vi "Base GEA3 Tool.vi"() -> ()   [LabVIEW 2021]
uses:
  Common/LabVIEW GEA2 Toolkit/GEA3/type defs/Data In.ctl
  Common/LabVIEW GEA2 Toolkit/GEA3/type defs/Source_Destination.ctl
  Common/LabVIEW GEA2 Toolkit/GEA3/type defs/ERD Write Data In.ctl
  Common/LabVIEW GEA2 Toolkit/GEA3/type defs/Data Type.ctl
  Common/LabVIEW GEA2 Toolkit/GEA3/type defs/ERD Read Data Out.ctl
  Common/LabVIEW GEA2 Toolkit/GEA3/type defs/ERD Read Data In.ctl
  Dryer Tool (Commercial 2)/JL Dryer Tool Support/type defs/Programming.ctl
  Dryer Tool (Commercial 2)/JL Dryer Tool Support/type defs/Flash_Results.ctl
  Dryer Tool (Commercial 2)/JL Dryer Tool Support/type defs/ERD_Always_Show_JL.ctl
  Common/GEA2 Script/typedefs/Script Info.ctl
  <vilib>/Platform/fileVersionInfo.llb/FileVersionInformation.ctl
  Dryer Tool (Commercial 2)/JL Dryer Tool Support/type defs/Choose_ERD_List.ctl
  Common/Diagnostics Decode/Type Defs/Diag_FaultTableStatus.ctl
  Common/Diagnostics Decode/Type Defs/Diag_FaultTableEntry.ctl
  Common/Diagnostics Decode/Type Defs/Diag_EntityManifestType.ctl
  Common/Diagnostics Decode/Type Defs/Diag_FaultSeqEntry.ctl
  Automation2/Product Specific/Clothes Care/Justice League/Product Testcode/Diagnostics/TypeDefs/Centauro Diagnostic V3 SnapShot.ctl
  Dryer Tool (Commercial 2)/JL Dryer Tool Support/type defs/JL_Diagnost V3 Cycle History.ctl
  Dryer Tool (Commercial 2)/JL Dryer Tool Support/type defs/ERDList.ctl
  Dryer Tool (Commercial 2)/JL Dryer Tool Support/type defs/ERD_Loop_States_JL.ctl
  Dryer Tool (Commercial 2)/JL Dryer Tool Support/type defs/Version.ctl
  Dryer Tool (Commercial 2)/JL Dryer Tool Support/type defs/BootloaderVersion.ctl
  Common/LabVIEW GEA2 Toolkit/GEA3/type defs/Data Out.ctl
  D:/Common/LabVIEW GEA2 Toolkit/source/GEA3 DLL Source/GeaCommunication.dll
  Common/LabVIEW GEA2 Toolkit/source/GEA3 DLL Source/GeaCommunication.dll
  Common/GExplorer Support/typedefs/GExplorer_Data_Cluster.ctl
  Dryer Tool (Commercial 2)/JL Dryer Tool Support/type defs/ERD_Data_Loop_Control.ctl
  Dryer Tool (Commercial 2)/JL Dryer Tool Support/type defs/Error_Command.ctl
  Dryer Tool (Commercial 2)/JL Dryer Tool Support/type defs/Cont_Send_States.ctl
  Dryer Tool (Commercial 2)/JL Dryer Tool Support/type defs/All_Bundled_Data_JL.ctl
  Dryer Tool (Commercial 2)/JL Dryer Tool Support/type defs/CSV_File_String_Arrays.ctl
  Dryer Tool (Commercial 2)/JL Dryer Tool Support/type defs/Fault Table Array.ctl
  Dryer Tool (Commercial 2)/JL Dryer Tool Support/type defs/Fault_Table_Info.ctl
  Dryer Tool (Commercial 2)/JL Dryer Tool Support/type defs/Heat Control.ctl
  Dryer Tool (Commercial 2)/JL Dryer Tool Support/type defs/ERD_Commercial_Laundry.ctl
  Dryer Tool (Commercial 2)/JL Dryer Tool Support/type defs/ERD_RJ45.ctl
  Dryer Tool (Commercial 2)/JL Dryer Tool Support/type defs/DAQ_Control_Command.ctl
  Dryer Tool (Commercial 2)/JL Dryer Tool Support/type defs/ERD_Loop_Control_Command.ctl
  Dryer Tool (Commercial 2)/JL Dryer Tool Support/type defs/GEA2_Control_Command.ctl
  Common/LabVIEW GEA2 Toolkit/GEA3/advanced/GEA2 Message Received Event Handler.vi
  Common/LabVIEW GEA2 Toolkit/GEA3/library/GEA2_Toolkit.lvlib
panel:
  out "Message":string
  in  "EndOfCycle":bool
  in  "Board Index":u8=1 min=3 max=10 step=1
  in  "Pause(mls)":u32=100
  out "Rate":u32=100
  out "State":T1=enum."Read ERDs"
  out "ERD_Always Show":T2={"Inlet Thermistor"=0, "Machine State"="IDLE", "Filtered Moisture"=0, "Cycle Selected"="", "HTR 1 / Inner / Top"=FALSE, "HTR 2 / Outer / Bot"=FALSE, "Door Switch"=FALSE, "Drum Light"=FALSE, "Cycle Engine State"="", "Centrifugal Switch"=FALSE, "Drum Motor"=FALSE, "Cycle Count"=0, "Ext. Tumble"=FALSE, "eDry"=FALSE, "Temp Level"="", "Dryness Level"="", "Time Level"="", "Delay Time (min)"=0, "Steam Refresh"=FALSE, "Damp Alert"=FALSE, "Sub-Cycle"="", "Outlet Thermistor"=0, "Target Moisture"=0, "Remaining Cycle Time"=0, "Raw Moisture"=0, "Cycle Name"="", "My Cycle"=FALSE, "Delay Dry"=FALSE, "Detangle"=FALSE, "Control Lock"=FALSE, "Steam Valve"=FALSE, "Door Latch"=FALSE, "Signal Volume"="", "Tune ID"="", "Restr Detect Status"="", "Vent Restriction"="", "Load Size by Contact"="", "Load Size by Temp"="", "EOC Reason"="", "Sensor Dry Status"="", "Dampness State"="", "Target Voltage Reached"=FALSE, "TrimInhibitR1"=FALSE, "TrimInhibitR2"=FALSE, "TrimBothCoilInhibit"=FALSE, "NormalHeatControl"=FALSE, "HeatControl Request"=FALSE, "Cool Down Status"="", "EcoDryInhibitRelay1"=FALSE, "EcoDryInhibitRelay2"=FALSE, "ReverseDrumInhibitRelay1"=FALSE, "ReverseDrumInhibitRelay2"=FALSE, "OverTempHeaterInhibitRequest"=FALSE, "FallbackHeatControlMethodStatus"=FALSE, "IHC TimeSeconds"=0, "ECT TimeSeconds "=0, "SC Total Drying Time(S')"=0, "TTR Target Voltage (S')"=0, "TCT Drying Time (S's)"=0, "Drum Motor State"=enum."Off", "Load Size by Ag"="", "MaxFIletered Voltage"=0, "Dry Load Detection"="", "Min Sensing Elapse Sec"=0, "Time Multi Sec X100"=0, "Time Adder  Sec"=0, "Temp Multi EcoDry"="", "Temp Multi ExtraLow"="", "Temp Multi Low "="", "Temp Multi Medium"="", "Temp Multi High"="", "SmoothMoisture"=0, "Eco Dry SEL Status"="", "Eco Dry SEL Result"="", "Eco Dry Cont Status"="", "Eco Dry Relay1 Timer"="", "Eco Dry Relay2 Timer "="", "Eco Dry Stage 2 Tans "=0, "WiFiCommissioningPSt"="IDLE", "Payment Method"=""}
  out "Temp ADC":T3
  in  "Read Parametric":bool=TRUE
  in  "Data ON":bool=TRUE
  in  "Stop":bool
  in  "Reset":bool
  in  "UI Launch":bool
  in  "Tab Control":T4(tab)=enum."ERD List"
  out "Personality Set":u8=1
  in  "?":u8=1
  in  "Set Personality":bool
  out "CSV File Log Path":path=path "D:/QA/Commercial 2/Dryer_Xolo/ProbandoC2_24-11-21_15-05-37.csv"
  out "Version":T5
  in  "Read ERD List":T6[](array[typedef])=[{"ERD Number"=49, "Data Type"=enum."string"}] {"ERD Number" format="%.0x"}
  in  "Read ERD":bool
  in  "Write ERD List":T7[](array[typedef])=[{"ERD Number"=49, "Data Type"=enum."string", "Data"="01"}] {"ERD Number" format="%.0x"}
  in  "Write ERD":bool
  out "Read ERD Data Out":T9[](array[typedef])=[{"ERD Number"=49, "Data"="00 00 00 16"}] {"ERD Number" format="%.0x"}
  out "Boot Loader Version":T10
  in  "GEA Inputs":T11={"Source"=229, "Destination"=192} {"Destination" format="%.0x"; "Source" format="%.0x"}
  out "OK?":bool
  in  "Parametric":T12(ring)
  in  "Exit Botloader":bool
  in  "Enum":enum16{"All", "MC", "UI"}(ring)
  in  "Entry Botloader":bool
  out "FileVersionInfo":T13
  out "LabView/Version Number":string
  in  "Tool Version":bool=TRUE
  out "GEA2 Log":string
  in  "Save Log":bool
  in  "GEA2 Log Length":i32=100000
  in  "Clear":bool
  in  "Ignore this CMD":string
  in  "Filter Data":bool=TRUE
  in  "Programming":T14={"Program"=FALSE, "File Path"=path "", "Program Ind"=FALSE, "Reset Board"=FALSE, "Enter Bootloader"=FALSE, "Result"=9} {"Result" items=["ImageRejected", "BoardNotFound", "UnableToGetGeaConfiguration", "WriteToFlashNotAllowed", "ImageDownloadedSuccessfully", "ImagePresent", "WriteToFlashFailed", "EraseFailed", "CrcFailed", ""]}
  in  "Flash Latest":bool
  in  "Send Button":bool
  in  "GEA2 Send":T16={"Source"=228, "Destination"=192, "Command"=0, "Message"=""} {"Command" format="%02x"; "Destination" format="%02x"; "Source" format="%02x"}
  in  "Msg Rate (ms)":u32=1000 min=50 step=50
  in  "Start Send":bool
  out "Converted Data Out":T17 {"CRC" format="%04x"; "Length" format="%02x"; "Command" format="%02x"; "Destination" format="%02x"; "Source" format="%02x"}
  in  "Write parametric":bool
  in  "Message to send":string="04 03"
  in  "Get Faults":bool
  in  "Clear Fault Table Buffer":bool
  in  "Clear Fault Seq Buffer":bool
  out "Fault Sequence Entries":T18[](array[typedef])
  out "Fault Seq Status":T19
  out "Fault Table Entries":T20[](array[typedef])
  out "Fault Table Status":T19
  out "Diagnostic Entity Manifest":T21
  out "Major Version":u8
  out "Minor Version":u8
  out "Fault Set?":bool
  in  "Filter by Count":bool=TRUE
  out "Centauro Fault Snapshot":T22
  in  "ERD Spam GEA Inputs":T11={"Source"=229, "Destination"=192} {"Destination" format="%.0x"; "Source" format="%.0x"}
  in  "Get Cycle Data":bool
  in  "Filter by Status Count":bool=TRUE
  out "JL Cycle History":T23
  out "output cluster":T19
  in  "Script Log Path":path
  in  "Run Script":bool
  out "Script Pass/Fail?":bool
  out "Script Report Text":string
  in  "stop script":bool
  in  "Script Path":path
  out "Script Info":T24 {"Overall Script File Progress" scale=0.0..1.0; "Elapsed time (s)" format="%#.1f"; "Current Script Progress" scale=0.0..1.0}
  out "Script Error Out":errorcluster
  in  "Load ERD List":T25
  in  "ERD Default List":T26 {"ERD Number" format="%x"}
  in  "ERD's List Ticket Testing":T26 {"ERD Number" format="%x"}
  in  "Wifi State":T27(ring)
  in  "Set Wifi State(ERD 6003)":bool
  in  "Turn on Wifi":bool
  in  "Turn off Wifi":bool
  out "Wifi Network State":string
  out "Wifi Password":string
  out "Wifi Network Name":string
  out "Mac Address":string
  in  "Get Wifi Data":bool
  out "Error Out":errorcluster
  # "Personality"
  # "Ver. 1.3"
  # "This controls destination of ERD Spam.\nYou should never change source unless\nyou want to see the spam in the GEA log."
  # "Wifi State is Writing to ERD 6003 and communicating with the wifi board directly.  It will remain in the state you wrote it to until another command is recieved. \n\nOnly Write to invalid if you are testing the board in Invalid state."
  # "After turning on Wifi , wait about 30 seconds and press the Get Wifi Data button.  Network state should be 1, apmode.\n\nAll this is doing is Writing the ERD 0xF115 Service Request to request connect, or disconnect."
  # "Contact:\n\nTerrance Bradford\nTerrance.Bradford@geappliances.com"
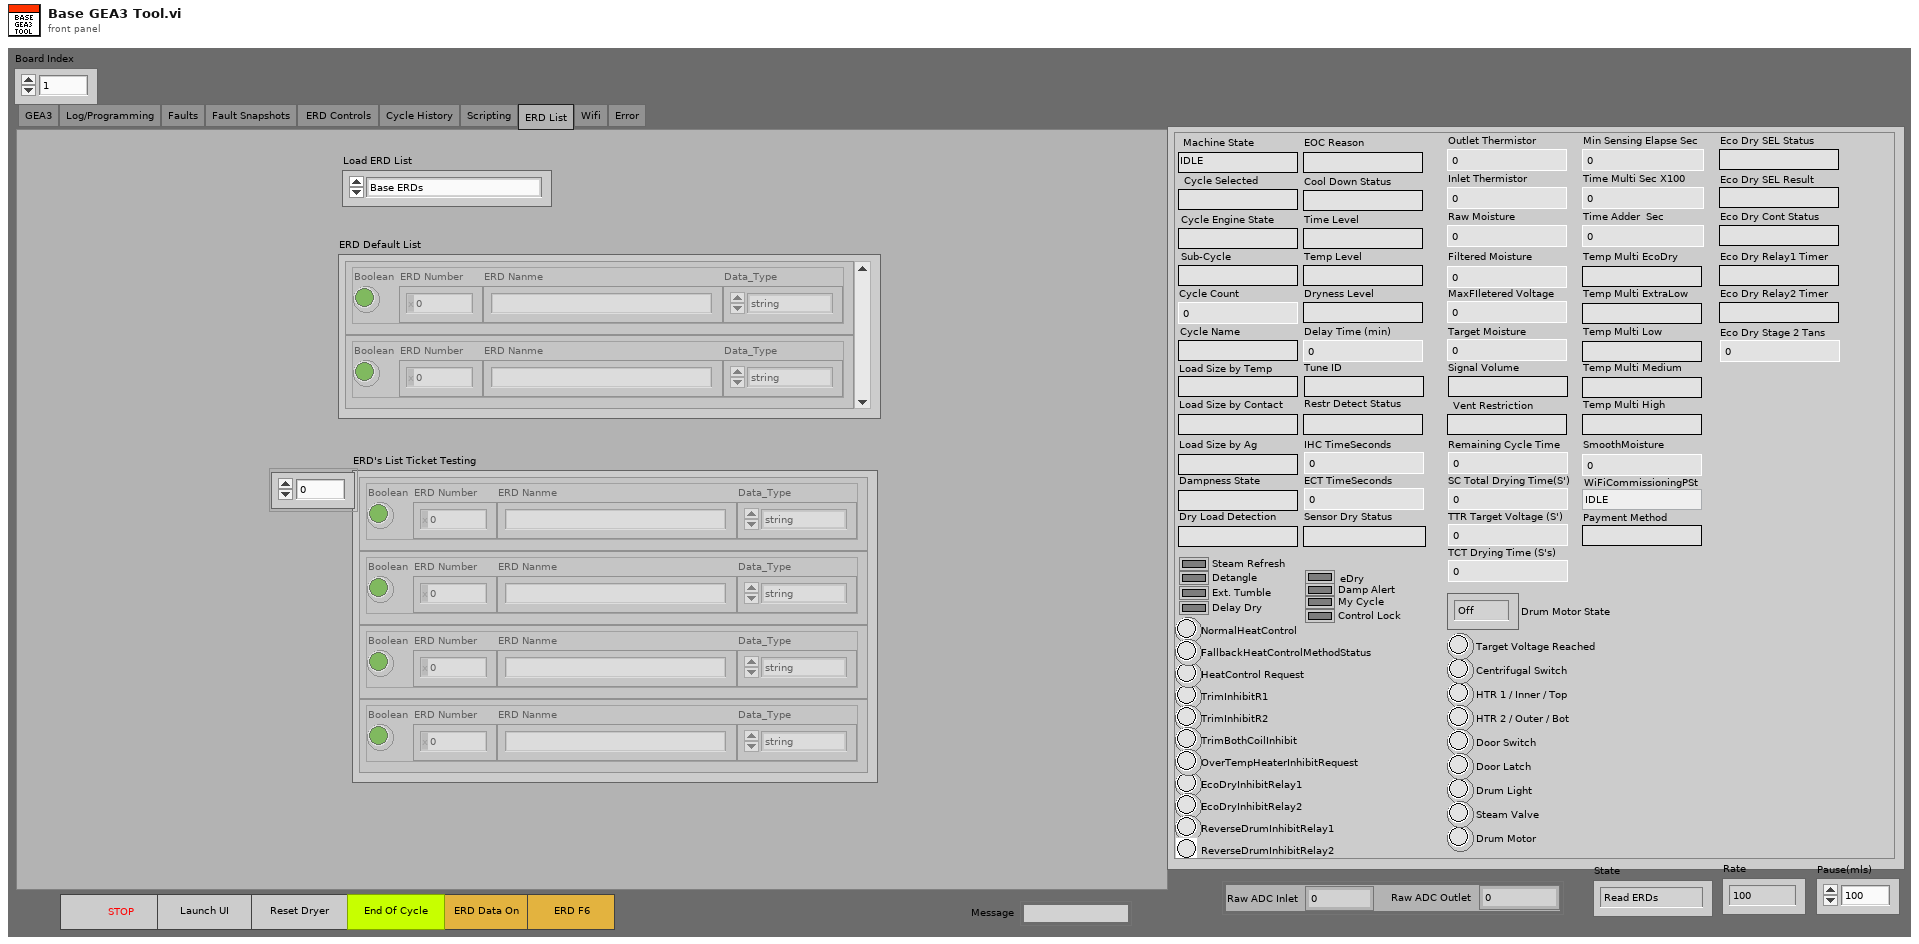
[diagram p1: front panel]
types:
  T1 = typedef "ERD_Loop_States_JL.ctl" = enum16{"Init", "Build ERD Read List", "Read ERDs", "Get Version", "ERD´s User show", "Update UI", "Read Faults", "Log Data", "Pause", "Shutdown"}
  T2 = typedef "ERD_Always_Show_JL.ctl" = cluster{"Inlet Thermistor":u16, "Machine State":string, "Filtered Moisture":u16, "Cycle Selected":string, "HTR 1 / Inner / Top":bool, "HTR 2 / Outer / Bot":bool, "Door Switch":bool, "Drum Light":bool, "Cycle Engine State":string, "Centrifugal Switch":bool, "Drum Motor":bool, "Cycle Count":u32, "Ext. Tumble":bool, "eDry":bool, "Temp Level":string, "Dryness Level":string, "Time Level":string, "Delay Time (min)":u16, "Steam Refresh":bool, "Damp Alert":bool, "Sub-Cycle":string, "Outlet Thermistor":u16, "Target Moisture":u16, "Remaining Cycle Time":u32, "Raw Moisture":u16, "Cycle Name":string, "My Cycle":bool, "Delay Dry":bool, "Detangle":bool, "Control Lock":bool, "Steam Valve":bool, "Door Latch":bool, "Signal Volume":string, "Tune ID":string, "Restr Detect Status":string, "Vent Restriction":string, "Load Size by Contact":string, "Load Size by Temp":string, "EOC Reason":string, "Sensor Dry Status":string, "Dampness State":string, "Target Voltage Reached":bool, "TrimInhibitR1":bool, "TrimInhibitR2":bool, "TrimBothCoilInhibit":bool, "NormalHeatControl":bool, "HeatControl Request":bool, "Cool Down Status":string, "EcoDryInhibitRelay1":bool, "EcoDryInhibitRelay2":bool, "ReverseDrumInhibitRelay1":bool, "ReverseDrumInhibitRelay2":bool, "OverTempHeaterInhibitRequest":bool, "FallbackHeatControlMethodStatus":bool, "IHC TimeSeconds":u32, "ECT TimeSeconds ":u32, "SC Total Drying Time(S')":u32, "TTR Target Voltage (S')":u32, "TCT Drying Time (S's)":u32, "Drum Motor State":enum16{"Off", "Cw", "Ccw", "Max"}, "Load Size by Ag":string, "MaxFIletered Voltage":u16, "Dry Load Detection":string, "Min Sensing Elapse Sec":u32, "Time Multi Sec X100":u32, "Time Adder  Sec":u32, "Temp Multi EcoDry":string, "Temp Multi ExtraLow":string, "Temp Multi Low ":string, "Temp Multi Medium":string, "Temp Multi High":string, "SmoothMoisture":u16, "Eco Dry SEL Status":string, "Eco Dry SEL Result":string, "Eco Dry Cont Status":string, "Eco Dry Relay1 Timer":string, "Eco Dry Relay2 Timer ":string, "Eco Dry Stage 2 Tans ":u32, "WiFiCommissioningPSt":string, "Payment Method":string}
  T3 = cluster{"Raw ADC Outlet":u16, "Raw ADC Inlet":u16}
  T4 = enum32{"GEA3", "Log/Programming", "Faults", "Fault Snapshots", "ERD Controls ", "Cycle History", "Scripting", "ERD List", "Wifi", "Error"}
  T5 = typedef "Version.ctl" = cluster{"Build Number":string, "Build Hash ":string, "Application Version":string, "Parametric Version":string, "UI App Version":string}
  T6 = typedef "ERD Read Data In.ctl" = cluster{"ERD Number":u16, "Data Type":enum16{"string", "boolean", "uint8_t", "uint16_t", "uint32_t", "uint64_t", "int8_t", "int16_t", "int32_t", "int64_t"}}
  T7 = typedef "ERD Write Data In.ctl" = cluster{"ERD Number":u16, "Data Type":T8, "Data":string}
  T8 = typedef "Data Type.ctl" = enum16{"string", "boolean", "uint8_t", "uint16_t", "uint32_t", "uint64_t", "int8_t", "int16_t", "int32_t", "int64_t"}
  T9 = typedef "ERD Read Data Out.ctl" = cluster{"ERD Number":u16, "Data":string}
  T10 = typedef "BootloaderVersion.ctl" = cluster{"UI BL Version":string, "MC BL Version":string}
  T11 = typedef "Source_Destination.ctl" = cluster{"Source":u8, "Destination":u8}
  T12 = enum16{"Board SKU", "Board Serial Number", "Unit SKU", "Unit Serial Number"}
  T13 = typedef "FileVersionInformation.ctl" = cluster{"FileVersion":string, "ProductName":string, "InternalName":string, "CompanyName":string, "LegalCopyright":string, "FileDescription":string}
  T14 = typedef "Programming.ctl" = cluster{"Program":bool, "File Path":path, "Program Ind":bool, "Reset Board":bool, "Enter Bootloader":bool, "Result":T15}
  T15 = typedef "Flash_Results.ctl" = i32
  T16 = typedef "Data In.ctl" = cluster{"Source":u8, "Destination":u8, "Command":u8, "Message":string}
  T17 = typedef "Data Out.ctl" = cluster{"Source":u8, "Destination":u8, "Command":u8, "Length":u8, "CRC":u16, "Message":string}
  T18 = typedef "Diag_FaultSeqEntry.ctl" = cluster{"Cycle #":u32, "Time":u32, "F Code":string, "F Active":bool}
  T19 = typedef "Diag_FaultTableStatus.ctl" = cluster{"Cur Index":u16, "Count":u16, "Ov Cnt":u16}
  T20 = typedef "Diag_FaultTableEntry.ctl" = cluster{"Cycle #":u32, "Time":u32, "F Code":string, "F Count":u16, "F Active":bool}
  T21 = typedef "Diag_EntityManifestType.ctl" = cluster{"ID":u8, "Data Ver Maj":u8, "Data Ver Min":u8, "Fault Table?":bool, "Fault Table Snap?":bool, "Fault Seq?":bool, "Fault Seq Snap?":bool, "Cycle History Seq?":bool, "Fault Table Entry Count":u16, "Fault Seq Entry Count":u16, "Cycle History Entry Count":u16, "Cycle Count":u32, "Entity Run Time (Min)":u32}
  T22 = typedef "Centauro Diagnostic V3 SnapShot.ctl" = string[][]
  T23 = typedef "JL_Diagnost V3 Cycle History.ctl" = string[][]
  T24 = typedef "Script Info.ctl" = cluster{"Overall Script File Progress":dbl, "Current Script Progress":dbl, "Script":string, "Test":string, "Elapsed time (s)":dbl, "Done?":bool}
  T25 = typedef "Choose_ERD_List.ctl" = enum16{"Base ERDs", "QA ERDs", "MABE ERD List", "EcoDry Evaluation ERD List", "ClothDampnessCheck ERD List"}
  T26 = typedef "ERDList.ctl" = cluster{"Boolean":bool, "ERD Number":u16, "ERD Nanme":string, "Data_Type":enum16{"string", "boolean", "uint8_t", "uint16_t", "uint32_t", "uint64_t", "int8_t", "int16_t", "int32_t", "int64_t"}}[]
  T27 = enum16{"0 - OFF", "1 - App Mode", "2 - Connecting", "3 - Connected", "4 - Connected Off", "5 - Scanning", "6 - Reconnecting", "255 - Invalid"}
  T28 = typedef "All_Bundled_Data_JL.ctl" = cluster{"Version":T5, "ERD_Always Show":T2, "Personality Set":u8, "CSV File String Arrays":T29, "Fault Table Array ":T30, "Heat Control":T32, "Temp ADC":cluster{"Raw ADC Outlet":u16, "Raw ADC Inlet":u16}, "Commercial_Laundry":T33, "Boot Loader Version":T10, "RJ45":T34}
  T29 = typedef "CSV_File_String_Arrays.ctl" = cluster{"ERD Number Array":string[], "ERD Name Array":string[], "ERD Converted String Data":string[]}
  T30 = typedef "Fault Table Array.ctl" = T31[]
  T31 = typedef "Fault_Table_Info.ctl" = cluster{"Cycle Count":u32, " Runtime (min) ":u32, "Fault Status":string, "Fault ID":string, "Fault Count":u16}
  T32 = typedef "Heat Control.ctl" = cluster{"Htr1 InletLowLim":string, "Htr1 InletUpLim":string, "Htr1 OutletLowLim":string, "Htr1 OutletUpLim":string, "Htr1 FallBackON(s)":string, "Htr1 FallBackOFF(s)":string, "Htr1":bool, "Htr2 InletLowLim":string, "Htr2 InletUpLim":string, "Htr2 OutletLowLim":string, "Htr2 OutletUpLim":string, "Htr2 FallBackON(s)":string, "Htr2 FallBackOFF(s)":string, "Htr2":bool}
  T33 = typedef "ERD_Commercial_Laundry.ctl" = cluster{"Session":string, "Phase":string, "Appliance Type":string, "Cycle Selected":string, "Platform Type":string, "Retry Signal":string, "Session Ext":string, "Phase Ext":string, "Appliance Type Ext":string, "Cycle Selected Ext":string, "Platform Type Ext":string, "Retry Signal Ext":string}
  T34 = typedef "ERD_RJ45.ctl" = cluster{"Write Access Actual":string, "Write Access Request":string, "LockedAtLeastOnce":string}
  T35 = typedef "Cont_Send_States.ctl" = enum16{"Run", "Shutdown"}
  T36 = typedef "ERD_Data_Loop_Control.ctl" = cluster{"Data":variant, "State":T1}
  T37 = typedef "Error_Command.ctl" = enum16{"Initialize", "Handle Errors", "Report Errors"}
  T38 = typedef "GExplorer_Data_Cluster.ctl" = cluster{"Data":variant, "State":enum16{"Add to Log", "Clear", "Shutdown"}}
  T39 = enum8{"Enabled", "Disabled", "Disabled and Grayed Out"}
  T40 = enum16{"UI Application APL", "UI Parametric APL", "MC APL"}
  T41 = typedef "GEA2_Control_Command.ctl" = enum16{"Initialize", "Shutdown"}
  T42 = typedef "ERD_Loop_Control_Command.ctl" = enum16{"Initialize", "Shutdown"}
  T43 = typedef "DAQ_Control_Command.ctl" = enum16{"Initialize", "Shutdown", "Exit"}
  T44 = typedef "F6_ERD_Control.ctl" = cluster{"EcoDryEnabledFlag":string, "KeyCycleId":u8, "CycleType":string, "Time LVL option 5":u32, "Time LVL option 4":u32, "Time LVL option _3":u32, "Time LVL option _2":u32, "Time LVL option _1":u32, "Time LVL option _0":u32, "CoolDownTimeInSeconds":u32, "TimeAdjustTimeCycleMinimumTimeInSeconds":u32, "TimeAdjustTimeCycleMaximumTimeInSeconds":u32, "TimeAdjustTimeCycleStandardAdjustTimeInSeconds":u32, "TimeAdjustTimeCycleSlewAdjustTimeInSeconds":u32, "ExtendedTumbleTimeInSeconds":u32, "SanitizeMaxDryTimeInSeconds":u32, "TemperatureDefault Level":u8, "Temperature ecoDryDefualtLevel":u8, "DrynessDefault Level":u8, "DrynessDefault ecoDryDefualtLevel":u8, "TimeAdjust defaultLevel":u8, "TimeAdjust ecoDryDefualtLevel":u8, "TimeLevelDefault Level":u8, "TimeLevelDefault Eco Dry":u8, "EStarSensorDry Default Level":u8, "EStarSensorDry ecoDryDefaultLevel":u8, "EcoDryDefault Level":u8, "EcoDryDefault EcoDryDefaultLevel ":u8, "ExtendedTumble Default Level":u8, "ExtendedTumble  EcoDryDefaultLevel":u8, "Sanitize Default Level":u8, "Sanitize ecoDryDefualtLevel":u8, "MyCycleDefault Level":u8, "MyCycleDefault ecoDryDefualtLevel":u8, "StartPause Default Level":u8, "StartPause ecoDryDefualtLevel":u8, "Power Default Level":u8, "Power ecoDryDefualtLevel":u8, "KeyVolume Default Level":u8, "KeyVolume ecoDryDefualtLevel":u8, "AlertVolume Default Level":u8, "AlertVolume ecoDryDefualtLevel":u8, "ControlLock Default Level":u8, "ControlLock EecoDryDefualtLevel":u8, "HeatControlRelay1EcoDryParametricDataEntry\nHeatControlTemperatureLimit_InletLower":u16, "HeatControlRelay1EcoDryParametricDataEntry\nHeatControlTemperatureLimit_InletUpper":u16, "HeatControlRelay1EcoDryParametricDataEntry\nHeatControlTemperatureLimit_OutletLower":u16, "HeatControlRelay1EcoDryParametricDataEntry\nHeatControlTemperatureLimit_OutletUpper":u16, "HeatControlRelay1EcoDryParametricDataEntry\nonTimeInSeconds":u8, "HeatControlRelay1EcoDryParametricDataEntry\noffTimeInSeconds":u8, "HeatControlRelay1EcoDryParametric\nDataEntryChange ":bool, "HeatControlRelay2 EcoDryParametricDataEntry\nHeatControlTemperatureLimit_InletLower":u16, "HeatControlRelay2 EcoDryParametricDataEntry\nHeatControlTemperatureLimit_InletUpper ":u16, "HeatControlRelay2EcoDryParametricDataEntry\nHeatControlTemperatureLimit_OutletLower ":u16, "HeatControlRelay2EcoDryParametricDataEntry\nHeatControlTemperatureLimit_OutletUpper":u16, "HeatControlRelay2EcoDryParametricDataEntry\nonTimeInSeconds ":u8, "HeatControlRelay2EcoDryParametricDataEntry\noffTimeInSeconds ":u8, "HeatControlRelay2EcoDry\nParametricDataEntryChange":bool, "DampAlert Default Level":u8, "DampAlert ecoDryDefaultLevel":u8, "Detangle Default Level ":u8, "Detangle ecoDryDefaultLevel":u8, "DelayStart Default Level":u8, "DelayStart ecoDryDefaultLevel":u8, "CycleAllowsInventoryChangeChange":bool, "TemperatureAllowable":u8, "DrynessAllowable":u8, "TimeLevelAllowable":u8, "EcoDryAllowable":u8, "ExtendedTumbleAllowable":u8, "DampAlertAllowable":u8, "DetangleAllowable":u8, "DelayStartAllowable":u8, "SanitizeAllowable":u8, "MyCycleAllowable":u8, "TimeAdjustAllowable":u8, "Power Allowable":u8, "KeyVolumeAllowable":u8, "AlertVolumeAllowable":u8, "ControlLockAllowable":u8, "EStarSensorDryAllowable":string, "StartPauseAllowable":u8, "EcoDryStage1Heater2\nActiveSeconds":u32, "EcoDryStage2PeriodSeconds":u32, "EcoDryStage2Heater1\nActiveSeconds":u32, "EcoDryStage2Heater2\nActiveSeconds":u32, "EcoDryStage1Heater1\nActiveSeconds":u32, "EcoDryStage1PeriodSeconds":u32, "EcoDryStage2DurationSeconds":u32, "CoolDownAdaptiveTargetTemperature":u16}
  T45 = enum32{"invalid app kind", "Development System", "Run Time System", "Student Edition", "Embedded LabVIEW", "Evaluation", "Custom"}
  T46 = typedef "eventsource.ctl" = u32
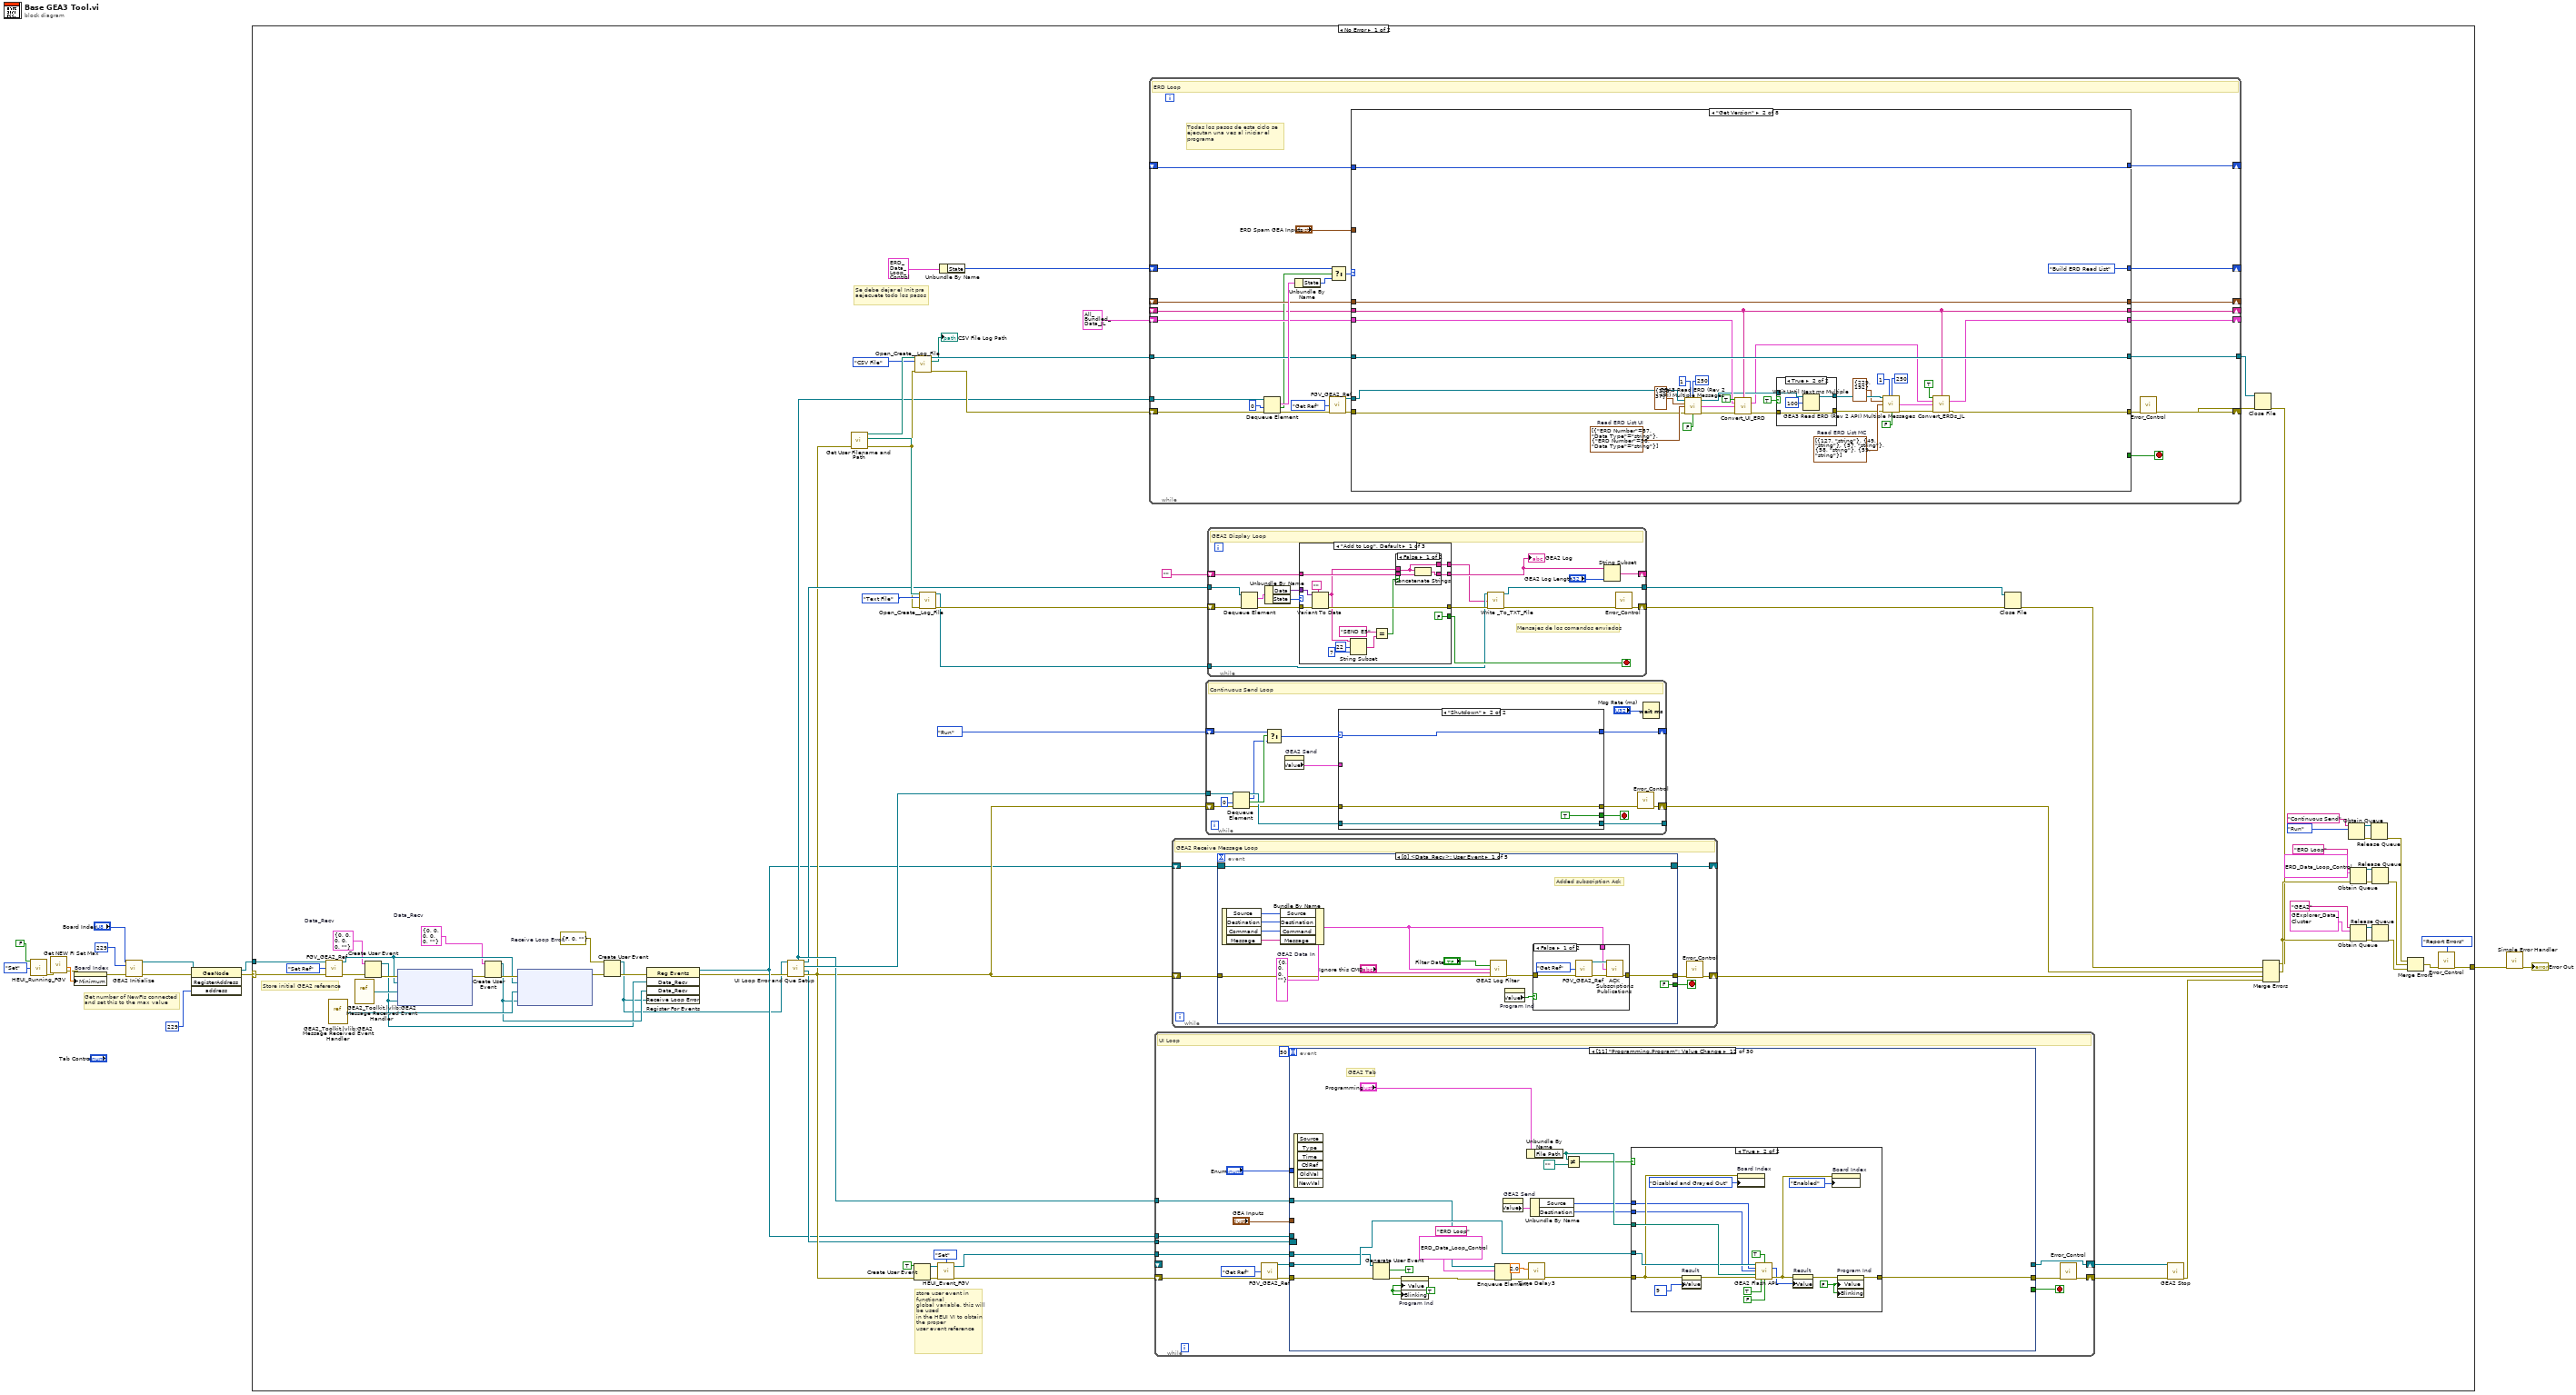
[diagram p0: block diagram]
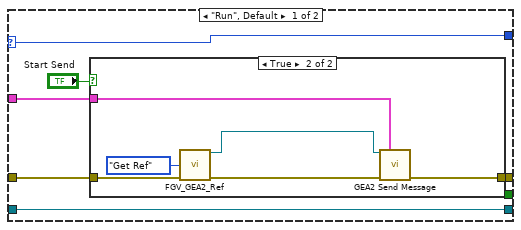
[diagram p2: hidden frame]
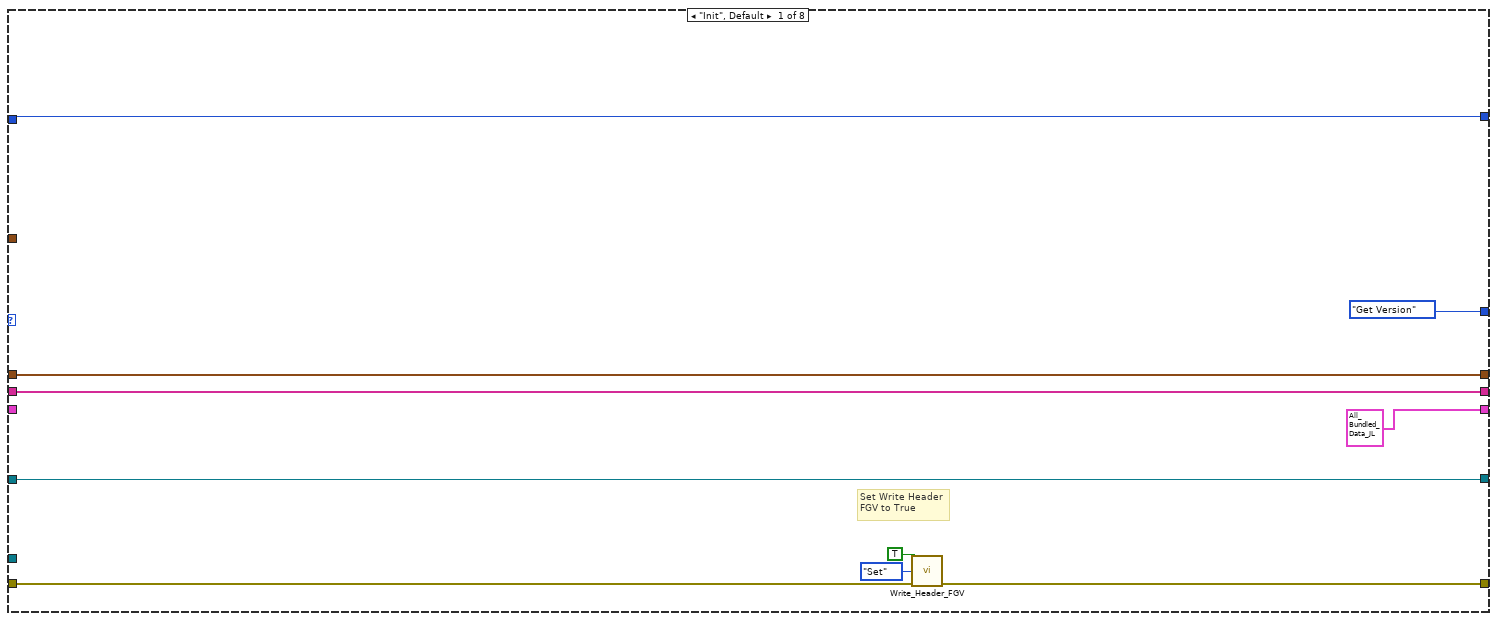
[diagram p4: hidden frame]
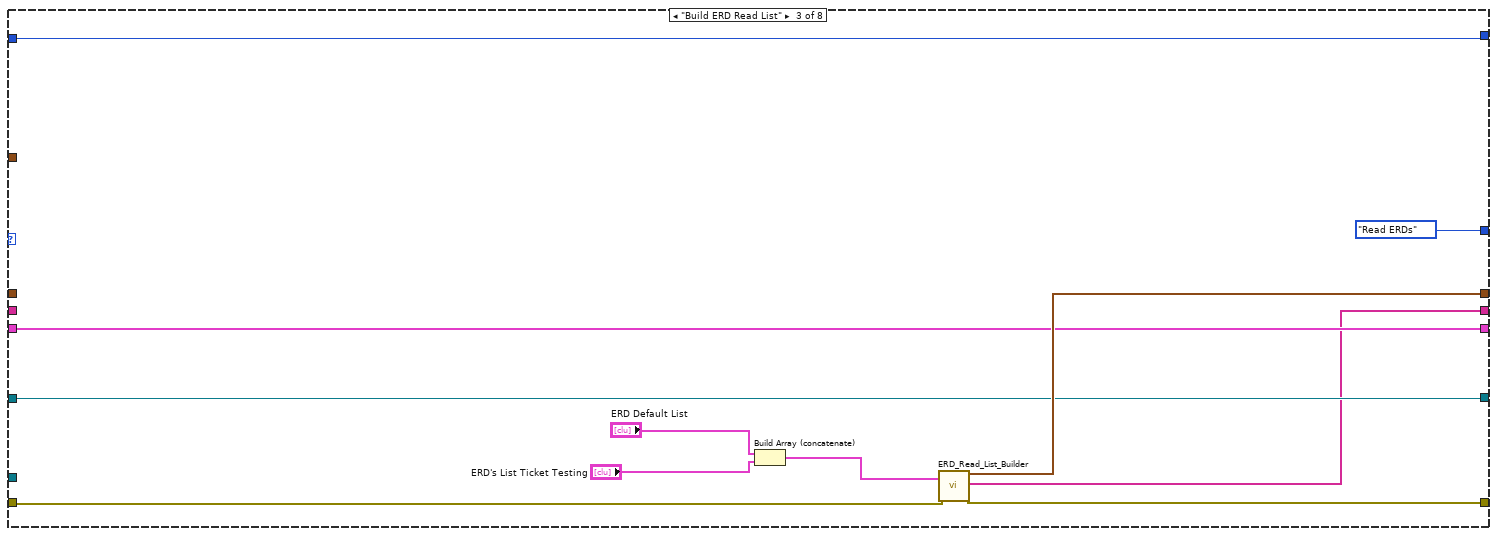
[diagram p6: hidden frame]
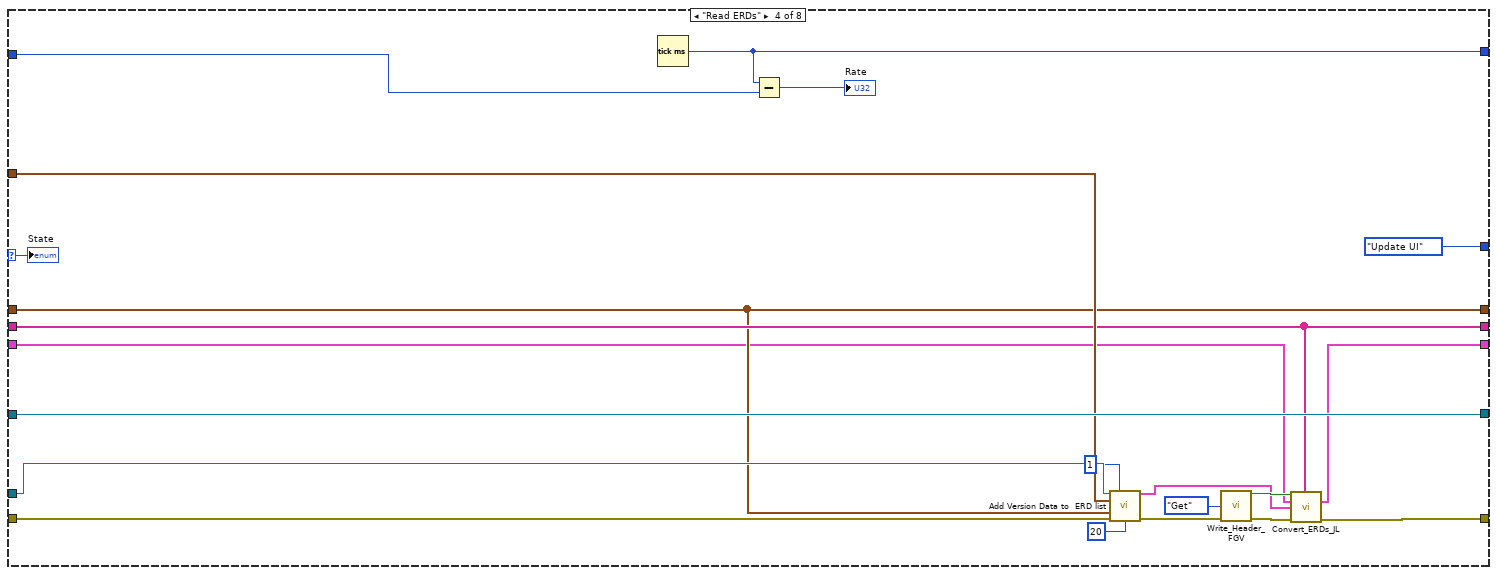
[diagram p7: hidden frame]
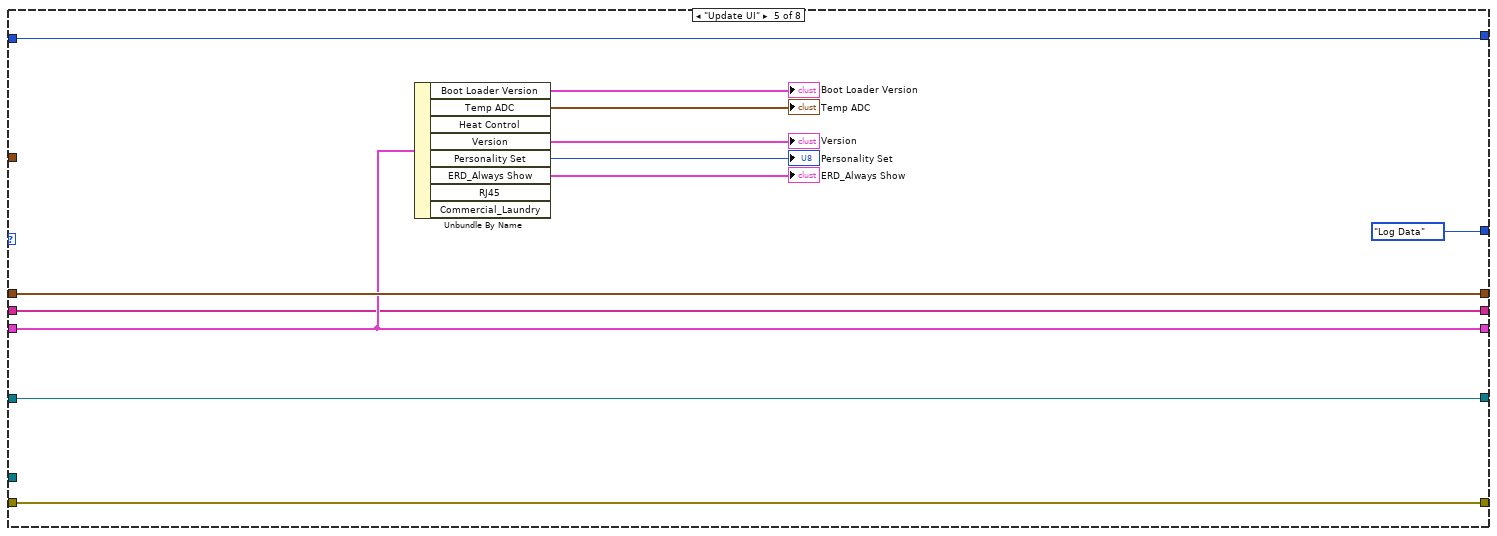
[diagram p8: hidden frame]
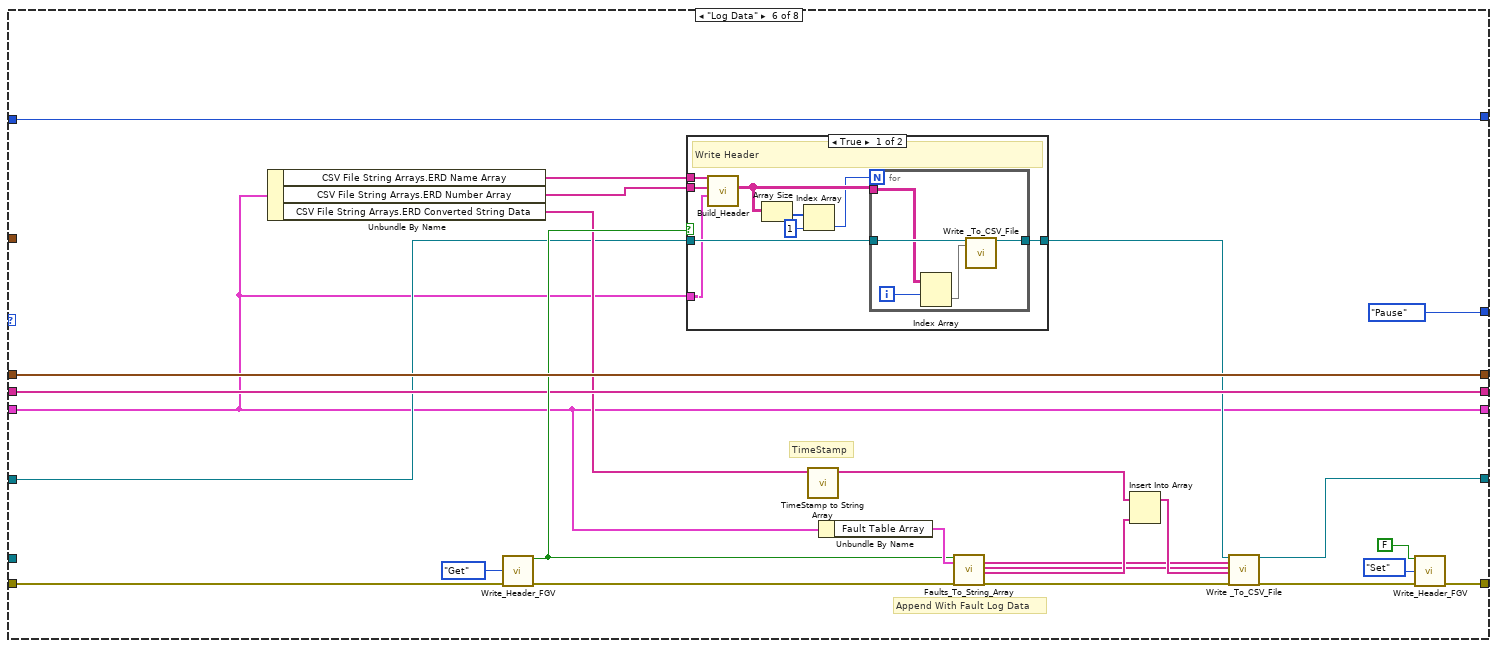
[diagram p9: hidden frame]
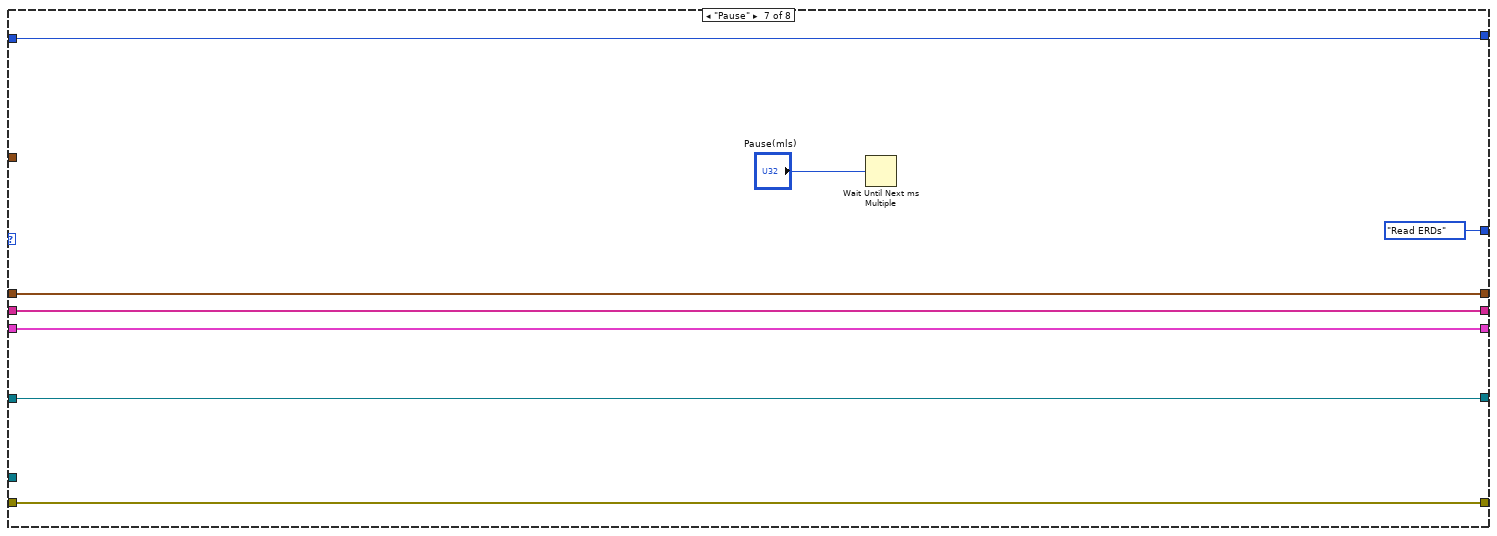
[diagram p11: hidden frame]
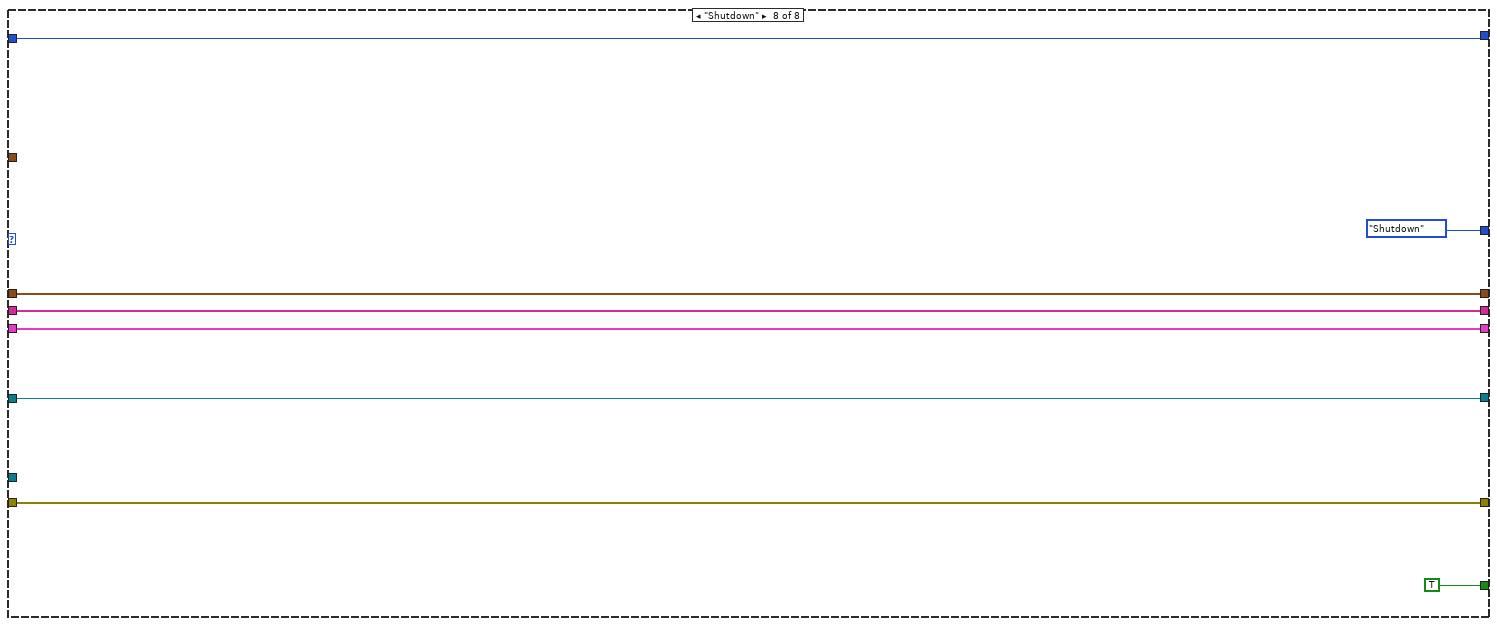
[diagram p12: hidden frame]
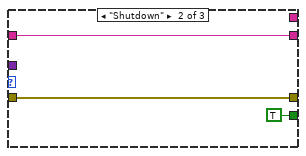
[diagram p14: hidden frame]
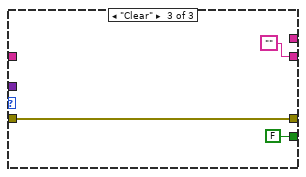
[diagram p15: hidden frame]
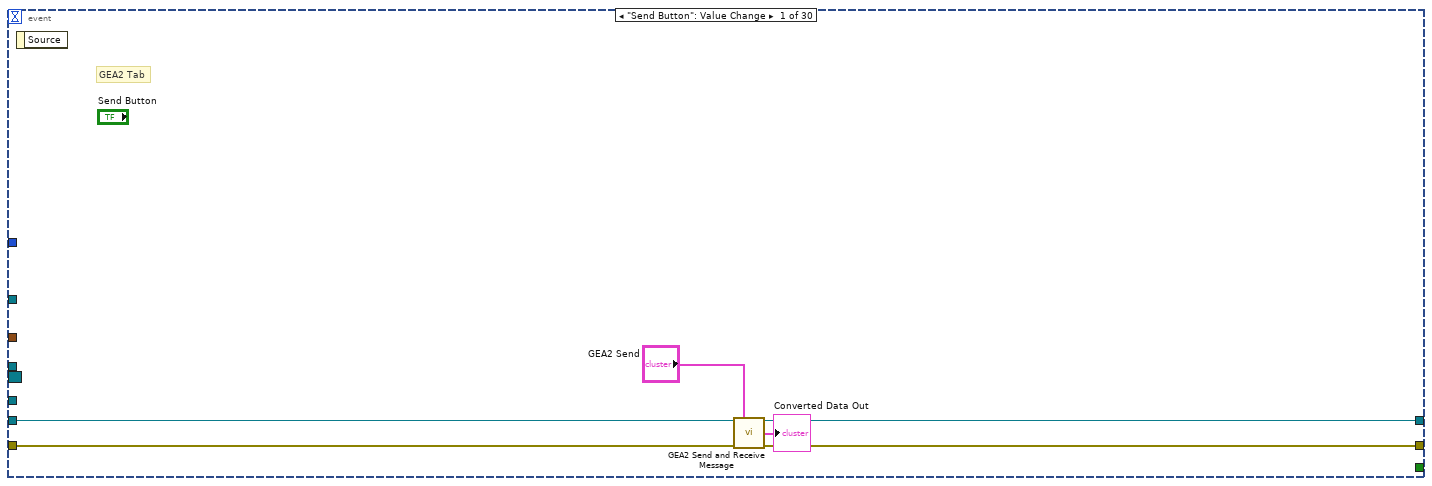
[diagram p16: hidden frame]
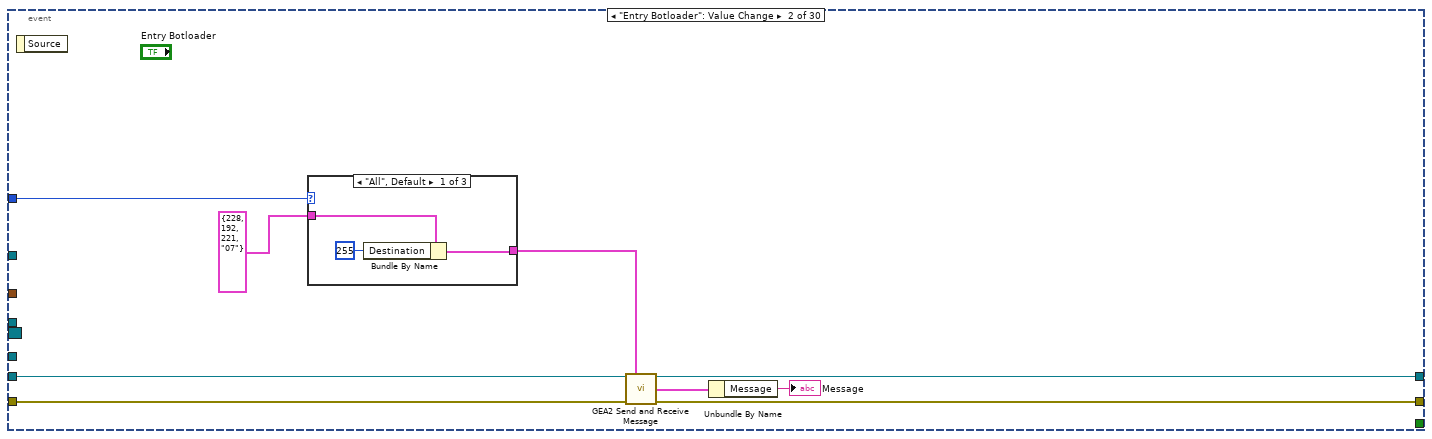
[diagram p17: hidden frame]
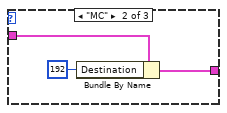
[diagram p18: hidden frame]
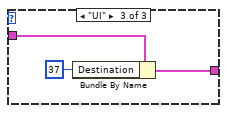
[diagram p19: hidden frame]
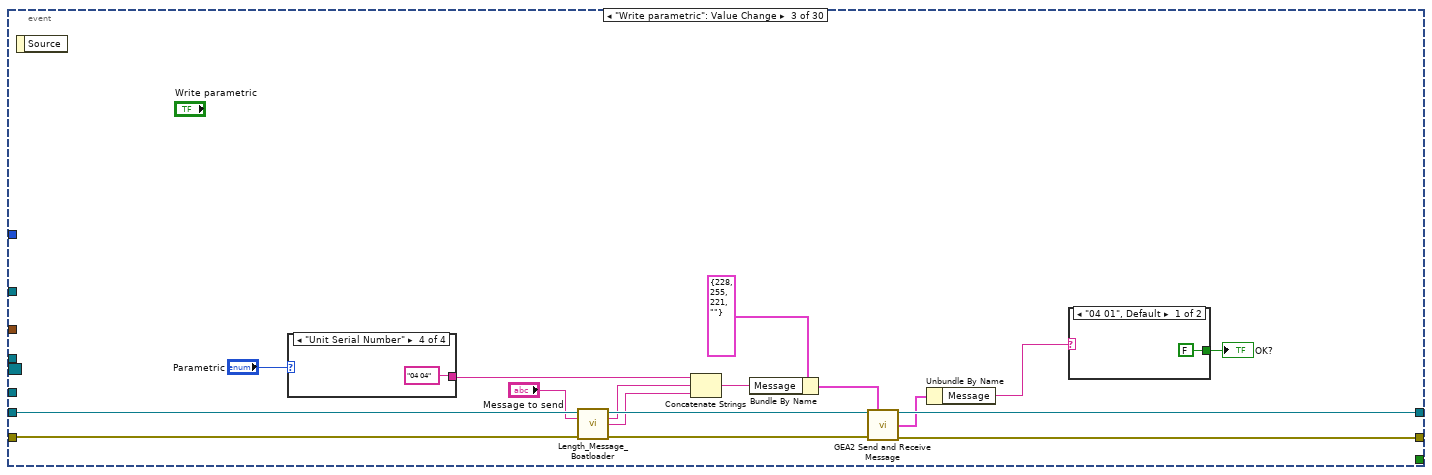
[diagram p20: hidden frame]
diagram:
  # "Get number of NewFIs connected\nand set this to the max value"
  n1 = call "HEUI_Running_FGV.vi"("Running?"=FALSE, "Action"=enum16{"Get", "Set"}."Set") -> ("Error Out"=w13:errorcluster)  [unwired: 12 in, 1 out]
  n2 = call "Get NEW FI Set Max.vi"("error in (no error)"=w13) -> ("Error Out"=w8:errorcluster, "Get Max_Out"=w9:dbl)  [unwired: 9 in]
  n3 = property on="Board Index" class="DigNum (strict)"(error in=w8, "Minimum"=w9) -> (error out=w7:errorcluster)  [unwired: 1 in, 1 out]
  n4 = call "GEA2 Initialize.vi"("Board Index"="Board Index", "Source Address"=u8 229, "error in"=w7) -> ("GEA2 Reference Out"=w5:refnum<k24>, "error out"=w2:errorcluster)  [unwired: 10 in, 1 out]
  n5 = invoke class="GeaNode" method="RegisterAddress"(reference=w5, error in=w2, "address"=u8 229 ("Source Address")) -> (reference out=w3:refnum<k24>, error out=w4:errorcluster)  [unwired: 1 in, 2 out]
  n6 = case shown="No Error" w4 {
    selector: w4 -> [w72 w977]
    tunnel: [w73 w977] -> w15
    tunnel: w3 -> [w36 _]
    frame No Error {
      w17 = T17 {"Source"=0, "Destination"=0, "Command"=0, "Length"=0, "CRC"=0, "Message"=""}  # Data_Recv
      w19 = T17 {"Source"=0, "Destination"=0, "Command"=0, "Length"=0, "CRC"=0, "Message"=""}  # Data_Recv
      w27 = errorcluster {"status"=FALSE, "code"=0, "source"=""}  # Receive Loop Error
      # "Se debe dejar el Init pra aejecuete todo los pasos"
      # "store user event in functional\nglobal variable, this will be used\nin the HEUI VI to obtain the proper\nuser event reference"
      # "Store initial GEA2 reference"
      n7 = call "FGV_GEA2_Ref.vi"("GEA2 Reference In"=w36, "Action"=enum16{"Set Ref", "Get Ref"}."Set Ref", "Error In"=w72) -> ("GEA2 Reference Out"=w30:refnum<k24>, "Error Out"=w18:errorcluster)  [unwired: 11 in]
      n8 = vi-ref "GEA2_Toolkit.lvlib:GEA2 Message Received Event Handler.vi"() -> (w28:refnum<vi>)
      n9 = vi-ref "GEA2_Toolkit.lvlib:GEA2 Message Received Event Handler.vi"() -> (w29:refnum<vi>)
      n10 = Create User Event(user event datatype=w19, error in=w18) -> (user event=w23:refnum<user-event>, error out=w32:errorcluster)
      n11 = node(w32, w30, w29, w23) -> (w33:errorcluster)  [unwired: 1 in, 1 out]
      n12 = Create User Event(user event datatype=w17, error in=w33) -> (user event=w24:refnum<user-event>, error out=w31:errorcluster)
      n13 = node(w31, w30, w28, w24) -> (w26:errorcluster)  [unwired: 1 in, 1 out]
      n14 = Create User Event(user event datatype=w27, error in=w26) -> (user event=w20:refnum<user-event>, error out=w25:errorcluster)
      n15 = register-events(error in=w25, w23, w24, w20) -> (reference out=w22:refnum<event-registration>, error out=w21:errorcluster)  [unwired: 1 in]
      n16 = call "UI Loop Error and Que Setup.vi"("error in (no error)"=w21, "Receive Loop"=w20) -> ("error out"=w37:errorcluster, "UI Loop Event Registration"=w35:refnum<event-registration>, "Continuous Send Queue"=w50:refnum<queue>, "GEA Display Queue"=w38:refnum<queue>, "ERD Queue Loop"=w39:refnum<queue>)  [unwired: 4 in, 1 out]
      n17 = call "Get User Filename and Path.vi"("error in (no error)"=w37) -> ("error out"=w40:errorcluster, "TXT File Path"=w46:path, "CSV File Path"=w48:path)  [unwired: 8 in]
      n18 = Create User Event(user event datatype=TRUE ("Bool"), error in=w37) -> (user event=w67:refnum<user-event>, error out=w68:errorcluster)
      n19 = call "Open_Create__Log_File.vi"("File Path Control"=w48, "Enum"=enum16{"CSV File", "Text File"}."CSV File", "Error In"=w40) -> ("refnum out"=w61:refnum<file>, "File Path"=→"CSV File Log Path":path, "Error Out"=w70:errorcluster)  [unwired: 10 in]
      n20 = call "Open_Create__Log_File.vi"("File Path Control"=w46, "Enum"=enum16{"CSV File", "Text File"}."Text File", "Error In"=w40) -> ("refnum out"=w45:refnum<file>, "Error Out"=w47:errorcluster)  [unwired: 10 in, 1 out]
      n21 = call "HEUI_Event_FGV.vi"("Event In"=w67, "Action"=enum16{"Get", "Set"}."Set", "Error In"=w68) -> ("Event Out"=w64:refnum<user-event>, "Error Out"=w65:errorcluster)  [unwired: 11 in]
      n22 = Unbundle By Name(T36 {"Data"=variant, "State"=enum."Init"} ("Data")) -> ("State"=w62:T1)
      n23 = while "Periodic ERD Query Loop" {
        shift-right: [w147] -> w59
        shift-left: w70 -> [w149]
        tunnel: w39 -> [w150]
        shift-right: [w141] -> _
        shift-left: w62 -> [w143]
        shift-right: [w136] -> _
        shift-left: _ -> [w135]
        tunnel: w61 -> [w134]
        tunnel: [w133] -> w57
        shift-right: [w132] -> _
        shift-left: T28 {"Version"={"Build Number"="", "Build Hash "="", "Application Version"="", "Parametric Version"="", "UI App Version"=""}, "ERD_Always Show"={"Inlet Thermistor"=0, "Machine State"="", "Filtered Moisture"=0, "Cycle Selected"="", "HTR 1 / Inner / Top"=FALSE, "HTR 2 / Outer / Bot"=FALSE, "Door Switch"=FALSE, "Drum Light"=FALSE, "Cycle Engine State"="", "Centrifugal Switch"=FALSE, "Drum Motor"=FALSE, "Cycle Count"=0, "Ext. Tumble"=FALSE, "eDry"=FALSE, "Temp Level"="", "Dryness Level"="", "Time Level"="", "Delay Time (min)"=0, "Steam Refresh"=FALSE, "Damp Alert"=FALSE, "Sub-Cycle"="", "Outlet Thermistor"=0, "Target Moisture"=0, "Remaining Cycle Time"=0, "Raw Moisture"=0, "Cycle Name"="", "My Cycle"=FALSE, "Delay Dry"=FALSE, "Detangle"=FALSE, "Control Lock"=FALSE, "Steam Valve"=FALSE, "Door Latch"=FALSE, "Signal Volume"="", "Tune ID"="", "Restr Detect Status"="", "Vent Restriction"="", "Load Size by Contact"="", "Load Size by Temp"="", "EOC Reason"="", "Sensor Dry Status"="", "Dampness State"="", "Target Voltage Reached"=FALSE, "TrimInhibitR1"=FALSE, "TrimInhibitR2"=FALSE, "TrimBothCoilInhibit"=FALSE, "NormalHeatControl"=FALSE, "HeatControl Request"=FALSE, "Cool Down Status"="", "EcoDryInhibitRelay1"=FALSE, "EcoDryInhibitRelay2"=FALSE, "ReverseDrumInhibitRelay1"=FALSE, "ReverseDrumInhibitRelay2"=FALSE, "OverTempHeaterInhibitRequest"=FALSE, "FallbackHeatControlMethodStatus"=FALSE, "IHC TimeSeconds"=0, "ECT TimeSeconds "=0, "SC Total Drying Time(S')"=0, "TTR Target Voltage (S')"=0, "TCT Drying Time (S's)"=0, "Drum Motor State"=enum."Off", "Load Size by Ag"="", "MaxFIletered Voltage"=0, "Dry Load Detection"="", "Min Sensing Elapse Sec"=0, "Time Multi Sec X100"=0, "Time Adder  Sec"=0, "Temp Multi EcoDry"="", "Temp Multi ExtraLow"="", "Temp Multi Low "="", "Temp Multi Medium"="", "Temp Multi High"="", "SmoothMoisture"=0, "Eco Dry SEL Status"="", "Eco Dry SEL Result"="", "Eco Dry Cont Status"="", "Eco Dry Relay1 Timer"="", "Eco Dry Relay2 Timer "="", "Eco Dry Stage 2 Tans "=0, "WiFiCommissioningPSt"="", "Payment Method"=""}, "Personality Set"=0, "CSV File String Arrays"={"ERD Number Array"=[], "ERD Name Array"=[], "ERD Converted String Data"=[]}, "Fault Table Array "=[], "Heat Control"={"Htr1 InletLowLim"="", "Htr1 InletUpLim"="", "Htr1 OutletLowLim"="", "Htr1 OutletUpLim"="", "Htr1 FallBackON(s)"="", "Htr1 FallBackOFF(s)"="", "Htr1"=FALSE, "Htr2 InletLowLim"="", "Htr2 InletUpLim"="", "Htr2 OutletLowLim"="", "Htr2 OutletUpLim"="", "Htr2 FallBackON(s)"="", "Htr2 FallBackOFF(s)"="", "Htr2"=FALSE}, "Temp ADC"={"Raw ADC Outlet"=0, "Raw ADC Inlet"=0}, "Commercial_Laundry"={"Session"="", "Phase"="", "Appliance Type"="", "Cycle Selected"="", "Platform Type"="", "Retry Signal"="", "Session Ext"="", "Phase Ext"="", "Appliance Type Ext"="", "Cycle Selected Ext"="", "Platform Type Ext"="", "Retry Signal Ext"=""}, "Boot Loader Version"={"UI BL Version"="", "MC BL Version"=""}, "RJ45"={"Write Access Actual"="", "Write Access Request"="", "LockedAtLeastOnce"=""}} ("All_ERD_Data_Bundled_Brass") -> [w131]
        shift-right: [w129] -> _
        shift-left: _ -> [w128]
        shift-right: [w126] -> _
        shift-left: _ -> [w125]
        stop <- w146 stop-if-true
        # "Todas los pasos de esta ciclo se ejecutan una ves al iniciar el programa"
        # "ERD Loop"
        n24 = Dequeue Element(queue=w150, timeout in ms (-1)=0, error in (no error)=w149) -> (element=w138:T36, timed out?=w130:bool, error out=w148:errorcluster)  [unwired: 1 out]
        n25 = Unbundle By Name(w138) -> ("State"=w144:T1)
        n26 = call "FGV_GEA2_Ref.vi"("Action"=enum16{"Set Ref", "Get Ref"}."Get Ref", "Error In"=w148) -> ("GEA2 Reference Out"=w137:refnum<k24>, "Error Out"=w140:errorcluster)  [unwired: 12 in]
        n27 = Select(t=w143, s=w130, f=w144) -> (s? t:f=w142:T1)
        n28 = case shown="\"Get Version\"" w142 {
          selector: w142 -> [_ _ _ w217 _ _ _ _]
          tunnel: w140 -> [w161 w169 w209 w220 w238 w264 w291 w299]
          tunnel: [w155 w187 w206 w225 w238 w261 w291 w299] -> w145
          tunnel: [_ _ _ _ _ _ _ TRUE] -> w146
          tunnel: "ERD Spam GEA Inputs" -> [_ _ _ w222 _ _ _ _]
          tunnel: [ERD_Loop_States_JL."Get Version" ("State") ERD_Loop_States_JL."Build ERD Read List" ("State") ERD_Loop_States_JL."Read ERDs" ("State") ERD_Loop_States_JL."Update UI" ("State") ERD_Loop_States_JL."Log Data" ("State") ERD_Loop_States_JL."Pause" ("t") ERD_Loop_States_JL."Read ERDs" ("State") ERD_Loop_States_JL."Shutdown" ("State")] -> w141
          tunnel: w137 -> [_ w170 _ w221 _ _ _ _]
          tunnel: [w159 w192 w208 w218 w241 w268 w289 w296] -> w136
          tunnel: w135 -> [w159 w192 _ w218 w241 w268 w289 w296]
          tunnel: w134 -> [w158 w191 w205 w229 w239 w249 w288 w295]
          tunnel: [w158 w191 w205 w229 w239 w267 w288 w295] -> w133
          tunnel: [T28 {"Version"={"Build Number"="", "Build Hash "="", "Application Version"="", "Parametric Version"="", "UI App Version"=""}, "ERD_Always Show"={"Inlet Thermistor"=0, "Machine State"="", "Filtered Moisture"=0, "Cycle Selected"="", "HTR 1 / Inner / Top"=FALSE, "HTR 2 / Outer / Bot"=FALSE, "Door Switch"=FALSE, "Drum Light"=FALSE, "Cycle Engine State"="", "Centrifugal Switch"=FALSE, "Drum Motor"=FALSE, "Cycle Count"=0, "Ext. Tumble"=FALSE, "eDry"=FALSE, "Temp Level"="", "Dryness Level"="", "Time Level"="", "Delay Time (min)"=0, "Steam Refresh"=FALSE, "Damp Alert"=FALSE, "Sub-Cycle"="", "Outlet Thermistor"=0, "Target Moisture"=0, "Remaining Cycle Time"=0, "Raw Moisture"=0, "Cycle Name"="", "My Cycle"=FALSE, "Delay Dry"=FALSE, "Detangle"=FALSE, "Control Lock"=FALSE, "Steam Valve"=FALSE, "Door Latch"=FALSE, "Signal Volume"="", "Tune ID"="", "Restr Detect Status"="", "Vent Restriction"="", "Load Size by Contact"="", "Load Size by Temp"="", "EOC Reason"="", "Sensor Dry Status"="", "Dampness State"="", "Target Voltage Reached"=FALSE, "TrimInhibitR1"=FALSE, "TrimInhibitR2"=FALSE, "TrimBothCoilInhibit"=FALSE, "NormalHeatControl"=FALSE, "HeatControl Request"=FALSE, "Cool Down Status"="", "EcoDryInhibitRelay1"=FALSE, "EcoDryInhibitRelay2"=FALSE, "ReverseDrumInhibitRelay1"=FALSE, "ReverseDrumInhibitRelay2"=FALSE, "OverTempHeaterInhibitRequest"=FALSE, "FallbackHeatControlMethodStatus"=FALSE, "IHC TimeSeconds"=0, "ECT TimeSeconds "=0, "SC Total Drying Time(S')"=0, "TTR Target Voltage (S')"=0, "TCT Drying Time (S's)"=0, "Drum Motor State"=enum."Off", "Load Size by Ag"="", "MaxFIletered Voltage"=0, "Dry Load Detection"="", "Min Sensing Elapse Sec"=0, "Time Multi Sec X100"=0, "Time Adder  Sec"=0, "Temp Multi EcoDry"="", "Temp Multi ExtraLow"="", "Temp Multi Low "="", "Temp Multi Medium"="", "Temp Multi High"="", "SmoothMoisture"=0, "Eco Dry SEL Status"="", "Eco Dry SEL Result"="", "Eco Dry Cont Status"="", "Eco Dry Relay1 Timer"="", "Eco Dry Relay2 Timer "="", "Eco Dry Stage 2 Tans "=0, "WiFiCommissioningPSt"="", "Payment Method"=""}, "Personality Set"=0, "CSV File String Arrays"={"ERD Number Array"=[], "ERD Name Array"=[], "ERD Converted String Data"=[]}, "Fault Table Array "=[], "Heat Control"={"Htr1 InletLowLim"="", "Htr1 InletUpLim"="", "Htr1 OutletLowLim"="", "Htr1 OutletUpLim"="", "Htr1 FallBackON(s)"="", "Htr1 FallBackOFF(s)"="", "Htr1"=FALSE, "Htr2 InletLowLim"="", "Htr2 InletUpLim"="", "Htr2 OutletLowLim"="", "Htr2 OutletUpLim"="", "Htr2 FallBackON(s)"="", "Htr2 FallBackOFF(s)"="", "Htr2"=FALSE}, "Temp ADC"={"Raw ADC Outlet"=0, "Raw ADC Inlet"=0}, "Commercial_Laundry"={"Session"="", "Phase"="", "Appliance Type"="", "Cycle Selected"="", "Platform Type"="", "Retry Signal"="", "Session Ext"="", "Phase Ext"="", "Appliance Type Ext"="", "Cycle Selected Ext"="", "Platform Type Ext"="", "Retry Signal Ext"=""}, "Boot Loader Version"={"UI BL Version"="", "MC BL Version"=""}, "RJ45"={"Write Access Actual"="", "Write Access Request"="", "LockedAtLeastOnce"=""}} ("All_ERD_Data_Bundled_Brass") w188 w204 w212 w240 w247 w287 w294] -> w132
          tunnel: w131 -> [_ w171 w204 w213 w240 w247 w287 w294]
          tunnel: [w154 w173 w203 w219 w235 w252 w286 w293] -> w129
          tunnel: w128 -> [w154 w173 _ w219 w235 w252 w286 w293]
          tunnel: [w153 w190 w202 w216 w234 w251 w285 w292] -> w126
          tunnel: w125 -> [w153 w190 w202 w215 w234 w251 w285 w292]
          frame "Init", Default {
            # "Set Write Header\nFGV to True"
            n29 = call "Write_Header_FGV.vi"("Write Header ? In"=TRUE, "Action"=enum16{"Get", "Set"}."Set", "Error In"=w161) -> ("Error Out"=w155:errorcluster)  [unwired: 11 in, 1 out]
          }
          frame "Get Version" {
            w178 = T6[] [{"ERD Number"=57, "Data Type"=enum."string"}, {"ERD Number"=58, "Data Type"=enum."string"}]  # Read ERD List UI
            w186 = T6[] [{"ERD Number"=127, "Data Type"=enum."string"}, {"ERD Number"=49, "Data Type"=enum."string"}, {"ERD Number"=57, "Data Type"=enum."string"}, {"ERD Number"=58, "Data Type"=enum."string"}, {"ERD Number"=59, "Data Type"=enum."string"}]  # Read ERD List MC
            n30 = call "GEA3 Read ERD (Rev 2 API) Multiple Messages.vi"("GEA2 Reference In"=w170, "Retry Count"=1 ("# of Iterations (Should be 2 except JL)"), "Read Timeout (ms)"=u32 250, "GEA Inputs"=cluster{"Source":u8, "Destination":u8} {"Source"=229, "Destination"=37}, "Read ERD List"=w178, "Error In"=w169, "Verify ERD Response?"=FALSE) -> ("GEA2 Reference Out"=w165:refnum<k24>, "ERD Data Out"=w174:cluster{"ERD Number":u16, "Data":string}[], "Error Out"=w176:errorcluster)  [unwired: 5 in, 1 out]
            n31 = call "Convert_UI_ERD.vi"("New Header?"=TRUE, "ERD Name"=w173, "ERD_Data_Bundled_Out"=w171, "Array"=w174, "Error In"=w176) -> ("All_ERD_Data_Bundled_Brass"=w163:T28, "Error Out"=w167:errorcluster)  [unwired: 9 in]
            n32 = case shown="True" TRUE {
              tunnel: [w194 w198] -> w168
              tunnel: w167 -> [w194 w198]
              tunnel: [w195 w197] -> w166
              tunnel: w165 -> [w195 w197]
              frame False {
              }
              frame True {
                n33 = Wait Until Next ms Multiple(millisecond multiple=u32 100) -> ()  [unwired: 1 out]
              }
            }
            n34 = call "GEA3 Read ERD (Rev 2 API) Multiple Messages.vi"("GEA2 Reference In"=w166, "Retry Count"=1 ("# of Iterations (Should be 2 except JL)"), "Read Timeout (ms)"=u32 250, "GEA Inputs"=cluster{"Source":u8, "Destination":u8} {"Source"=229, "Destination"=192}, "Read ERD List"=w186, "Error In"=w168, "Verify ERD Response?"=FALSE) -> ("ERD Data Out"=w175:cluster{"ERD Number":u16, "Data":string}[], "Error Out"=w184:errorcluster)  [unwired: 5 in, 2 out]
            n35 = call "Convert_ERDs_JL.vi"("New Header?"=TRUE, "ERD Name"=w173, "ERD_Data_Bundled_Out"=w163, "Array"=w175, "Error In"=w184) -> ("All_ERD_Data_Bundled_Brass"=w188:T28, "Error Out"=w187:errorcluster)  [unwired: 9 in]
          }
          frame "Build ERD Read List" {
            n36 = Build Array (concatenate)("ERD Default List", "ERD's List Ticket Testing") -> (w200:T26)
            n37 = call "ERD_Read_List_Builder.vi"("ERD Read List ALL"=w200, "Error In"=w209) -> ("Read ERD List"=w208:T6[], "ERD Name"=w203:string[], "Error Out"=w206:errorcluster)  [unwired: 15 in]
          }
          frame "Read ERDs" {
            n38 = Tick Count (ms)() -> (millisecond timer value=w216:u32)
            n39 = Subtract(x=w216, y=w215) -> (x-y=→"Rate":u32)
            n40 = call "Add Version Data to  ERD list.vi"(".NET Refnum in"=w221, "# of Iterations (Should be 2 except JL)"=1, "GEA Inputs"=w222, "Read ERD List MC"=w218, "error in (no error)"=w220, "#ERDs per message"=20) -> ("ERD Data Out out"=w224:T9[], "error out"=w223:errorcluster)  [unwired: 8 in]
            n41 = call "Write_Header_FGV.vi"("Action"=enum16{"Get", "Set"}."Get", "Error In"=w223) -> ("Write Header ? Out"=w226:bool, "Error Out"=w228:errorcluster)  [unwired: 12 in]
            n42 = call "Convert_ERDs_JL.vi"("New Header?"=w226, "ERD Name"=w219, "ERD_Data_Bundled_Out"=w213, "Array"=w224, "Error In"=w228) -> ("All_ERD_Data_Bundled_Brass"=w212:T28, "Error Out"=w225:errorcluster)  [unwired: 9 in]
            "State" <- w217
          }
          frame "Update UI" {
            n43 = Unbundle By Name(w240) -> ("Boot Loader Version"=→"Boot Loader Version":T10, "Temp ADC"=→"Temp ADC":T3, "Version"=→"Version":T5, "Personality Set"=→"Personality Set":u8, "ERD_Always Show"=→"ERD_Always Show":T2)  [unwired: 3 out]
          }
          frame "Log Data" {
            # "TimeStamp"
            # "Append With Fault Log Data"
            n44 = Unbundle By Name(w247) -> ("CSV File String Arrays.ERD Name Array"=w266:string[], "CSV File String Arrays.ERD Number Array"=w243:string[], "CSV File String Arrays.ERD Converted String Data"=w250:string[])
            n45 = call "Write_Header_FGV.vi"("Action"=enum16{"Get", "Set"}."Get", "Error In"=w264) -> ("Write Header ? Out"=w253:bool, "Error Out"=w259:errorcluster)  [unwired: 12 in]
            n46 = case shown="True" w253 {
              tunnel: w266 -> [w277 _]
              tunnel: w249 -> [w276 w283]
              tunnel: [w275 w283] -> w248
              tunnel: w247 -> [w274 _]
              tunnel: w243 -> [w273 _]
              frame True {
                # "Write Header"
                n47 = call "Build_Header.vi"("All_ERD_Data_Bundled_Brass out"=w274, "ERD Number Array In"=w273, "ERD Name Array In"=w277) -> ("ERD Name Array out 2"=w272:string[][])  [unwired: 8 in]
                n48 = Array Size(array=w272) -> (size(s)=w271:i32[])
                n49 = Index Array(array=w271, index=1) -> (element=w269:i32)
                n50 = for {
                  N: w269 -> [_]
                  tunnel: w276 -> [w282]
                  tunnel: [w281] -> w275
                  tunnel: w272 -> [w280]
                  i -> [w279]
                  n51 = Index Array(array=w280, index (row)=w279) -> (element=w278:string[])  [unwired: 1 in]
                  n52 = call "Write _To_CSV_File.vi"("Refnum In"=w282, "ERD Name"=w278) -> ("Refnum Out"=w281:refnum<file>)  [unwired: 15 in, 2 out]
                }
              }
              frame False {
              }
            }
            n53 = call "TimeStamp to String Array.vi"("String Array In"=w250) -> ("String Array Out"=w246:string[])  [unwired: 10 in]
            n54 = Unbundle By Name(w247) -> ("Fault Table Array"=w255:T30)
            n55 = call "Faults_To_String_Array.vi"("Write Header ?"=w253, "Fault Table Entry"=w255, "Error In"=w259) -> ("Fault Header String Array"=w245:string[], "Fault ERD Number String Array"=w244:string[], "Fault Data String Array"=w258:string[], "Error Out"=w256:errorcluster)  [unwired: 13 in]
            n56 = Insert Into Array(array=w246, new element=w258) -> (w257:string[])  [unwired: 1 in]
            n57 = call "Write _To_CSV_File.vi"("Refnum In"=w248, "ERD Name"=w245, "ERD Number"=w244, "ERD Data"=w257, "Error In"=w256) -> ("Refnum Out"=w267:refnum<file>, "Error Out"=w262:errorcluster)  [unwired: 12 in, 1 out]
            n58 = call "Write_Header_FGV.vi"("Write Header ? In"=FALSE, "Action"=enum16{"Get", "Set"}."Set", "Error In"=w262) -> ("Error Out"=w261:errorcluster)  [unwired: 11 in, 1 out]
          }
          frame "Pause" {
            n59 = Wait Until Next ms Multiple(millisecond multiple="Pause(mls)") -> ()  [unwired: 1 out]
          }
          frame "Shutdown" {
          }
        }
        n60 = call "Error_Control.vi"("Error In"=w145) -> ("Error Out"=w147:errorcluster)  [unwired: 14 in]
      }
      n61 = while "UI Loop" {
        shift-right: [w353] -> w90
        shift-left: w65 -> [w347]
        shift-right: [w355] -> w89
        shift-left: _ -> [_]
        tunnel: w35 -> [w354]
        tunnel: w64 -> [w344]
        tunnel: w39 -> [w343]
        tunnel: w22 -> [w342]
        stop <- w352 stop-if-true
        # "UI Loop"
        n62 = call "FGV_GEA2_Ref.vi"("Action"=enum16{"Set Ref", "Get Ref"}."Get Ref", "Error In"=w347) -> ("GEA2 Reference Out"=w346:refnum<k24>, "Error Out"=w348:errorcluster)  [unwired: 12 in]
        n63 = event shown="[11] \"Programming.Program\": Value Change" {
          selector: w354 -> [_ _ _ _ _ _ _ _ _ _ _ _ _ _ _ _ _ _ _ _ _ _ _ _ _ _ _ _ _ _]
          dyn-events: _ -> [_ _ _ _ _ _ _ _ _ _ _ _ _ _ _ _ _ _ _ _ _ _ _ _ _ _ _ _ _ _]
          timeout: 50 -> [_ _ _ _ _ _ _ _ _ _ _ _ _ _ _ _ _ _ _ _ _ _ _ _ _ _ _ _ _ _]
          tunnel: [w358 w367 w394 w403 w424 w430 w442 w446 w453 w468 w481 w494 w537 w590 w596 w614 w617 w631 w680 w687 w702 w734 w750 w778 w789 w802 w813 _ w869 w876] -> w351
          tunnel: w348 -> [w359 w369 w387 w406 w421 w428 w442 w447 w452 w467 w488 w502 w542 w595 w606 w612 w621 w628 w678 w688 w703 w735 w747 w779 w797 w802 w820 w826 w873 w878]
          tunnel: [_ _ _ _ _ _ _ _ _ _ _ _ _ _ _ _ _ _ _ _ _ _ _ _ TRUE _ _ _ _ _] -> w352
          tunnel: w346 -> [w360 w370 w393 w405 w423 w434 w443 w450 w456 _ w487 w503 w543 w594 w605 w610 _ w640 _ w685 w700 w738 w748 _ w800 w803 w819 w827 w874 w877]
          tunnel: [w361 w368 w395 w404 w423 _ w443 w451 w457 _ w486 _ _ _ w604 w608 _ _ _ w686 w701 w736 w749 _ w800 w803 w814 _ w870 w875] -> w355
          tunnel: "GEA Inputs" -> [_ _ _ _ _ w433 _ w449 w455 _ w485 _ _ _ _ w609 _ _ _ w684 w704 w737 w751 _ _ _ _ w828 w871 _]
          tunnel: w344 -> [_ _ _ _ _ _ _ _ _ _ _ w499 w541 _ _ _ _ w625 _ _ _ _ _ _ _ _ _ _ _ _]
          tunnel: w343 -> [_ _ _ _ _ w429 _ _ _ _ _ w493 w538 w589 _ w613 _ w626 w676 _ _ _ _ w776 w788 _ _ _ _ _]
          tunnel: w342 -> [_ _ _ _ _ _ _ _ _ _ _ _ _ _ _ _ _ _ _ _ _ _ _ _ _ _ _ _ _ _]
          tunnel: "Enum" -> [_ w362 _ w402 _ _ _ _ _ _ _ _ _ _ _ _ _ _ _ _ _ _ _ _ _ _ _ _ _ _]
          event "Send Button": Value Change {
            # "GEA2 Tab"
            n64 = event-data() -> ()  [unwired: 1 in, 1 out]
            n65 = call "GEA2 Send and Receive Message.vi"("GEA2 Reference In"=w360, "Input Data"="GEA2 Send", "Error In"=w359) -> ("GEA2 Reference Out"=w361:refnum<k24>, "Converted Data Out"=→"Converted Data Out":T17, "Error Out"=w358:errorcluster)  [unwired: 9 in, 1 out]
          }
          event "Entry Botloader": Value Change {
            n66 = event-data() -> ()  [unwired: 1 in, 1 out]
            n67 = case shown="\"All\", Default" w362 {
              tunnel: T16 {"Source"=228, "Destination"=192, "Command"=221, "Message"="07"} ("GEA2 Send") -> [w372 w376 w377]
              tunnel: [w371 w374 w378] -> w363
              frame "All", Default {
                n68 = Bundle By Name(cluster=w372, "Destination"=u8 255) -> (w371:T16)
              }
              frame "MC" {
                n69 = Bundle By Name(cluster=w376, "Destination"=u8 192) -> (w374:T16)
              }
              frame "UI" {
                n70 = Bundle By Name(cluster=w377, "Destination"=u8 37) -> (w378:T16)
              }
            }
            n71 = call "GEA2 Send and Receive Message.vi"("GEA2 Reference In"=w370, "Input Data"=w363, "Error In"=w369) -> ("GEA2 Reference Out"=w368:refnum<k24>, "Converted Data Out"=w366:T17, "Error Out"=w367:errorcluster)  [unwired: 9 in, 1 out]
            n72 = Unbundle By Name(w366) -> ("Message"=→"Message":string)
          }
          event "Write parametric": Value Change {
            n73 = event-data() -> ()  [unwired: 1 in, 1 out]
            n74 = case shown="\"Unit Serial Number\"" "Parametric" {
              tunnel: ["04 01" ("string") "04 02" ("string") "04 03" ("string") "04 04" ("string")] -> w391
              frame "Board SKU", Default {
              }
              frame "Board Serial Number" {
              }
              frame "Unit SKU" {
              }
              frame "Unit Serial Number" {
              }
            }
            n75 = call "Length_Message_Boatloader.vi"("string"="Message to send", "error in"=w387) -> ("hex integer string"=w389:string, "Message"=w388:string, "error out"=w386:errorcluster)  [unwired: 11 in]
            n76 = Concatenate Strings(w391, w389, w388) -> (w384:string)
            n77 = Bundle By Name(cluster=T16 {"Source"=228, "Destination"=255, "Command"=221, "Message"=""} ("GEA2 Send"), "Message"=w384) -> (w383:T16)
            n78 = call "GEA2 Send and Receive Message.vi"("GEA2 Reference In"=w393, "Input Data"=w383, "Error In"=w386) -> ("GEA2 Reference Out"=w395:refnum<k24>, "Converted Data Out"=w382:T17, "Error Out"=w394:errorcluster)  [unwired: 9 in, 1 out]
            n79 = Unbundle By Name(w382) -> ("Message"=w381:string)
            n80 = case shown="\"04 01\", Default" w381 {
              tunnel: [FALSE TRUE] -> w380
              frame "04 01", Default {
              }
              frame "04 00" {
              }
            }
            "OK?" <- w380
          }
          event "Exit Botloader": Value Change {
            n81 = event-data() -> ()  [unwired: 1 in, 1 out]
            n82 = case shown="\"All\", Default" w402 {
              tunnel: T16 {"Source"=228, "Destination"=0, "Command"=221, "Message"="F4 01"} ("GEA2 Send") -> [w410 w414 w415]
              tunnel: [w409 w412 w416] -> w407
              frame "All", Default {
                n83 = Bundle By Name(cluster=w410, "Destination"=u8 255) -> (w409:T16)
              }
              frame "MC" {
                n84 = Bundle By Name(cluster=w414, "Destination"=u8 192) -> (w412:T16)
              }
              frame "UI" {
                n85 = Bundle By Name(cluster=w415, "Destination"=u8 37) -> (w416:T16)
              }
            }
            n86 = call "GEA2 Send and Receive Message.vi"("GEA2 Reference In"=w405, "Input Data"=w407, "Error In"=w406) -> ("GEA2 Reference Out"=w404:refnum<k24>, "Error Out"=w403:errorcluster)  [unwired: 9 in, 2 out]
          }
          event "Clear": Value Change {
            w418 = T38 {"Data"=variant, "State"=enum."Clear"} ("element")
            # "GEA2 Tab"
            n87 = event-data() -> ()  [unwired: 1 in, 6 out]
            n88 = Obtain Queue(name (unnamed)="GEA2", element data type=w418, error in (no error)=w421) -> (queue out=w419:refnum<queue>, error out=w422:errorcluster)  [unwired: 2 in, 1 out]
            n89 = Enqueue Element(queue=w419, element=w418, error in (no error)=w422) -> (error out=w424:errorcluster)  [unwired: 1 in, 2 out]
          }
          event "Set Personality": Value Change {
            # "GEA2 Tab"
            n90 = event-data() -> ()  [unwired: 1 in, 6 out]
            n91 = Index Array(array=T7[] [{"ERD Number"=65281, "Data Type"=enum."string", "Data"=""}] ("Write ERD List")) -> (element=w439:T7)  [unwired: 1 in]
            n92 = Number To Hexadecimal String(1:i16 2 ("width (-)"), 2:"?") -> (0:w438:string)
            n93 = Bundle By Name(cluster=w439, "Data"=w438) -> (w437:T7)
            n94 = Build Array(w437) -> (w436:T7[])
            n95 = call "GEA2 Write ERD.vi"("GEA2 Reference In"=w434, "GEA Inputs"=w433, "Write ERD List"=w436, "Error In"=w428, "Verify ERD Response?"=TRUE) -> ("Error Out"=w426:errorcluster)  [unwired: 8 in, 2 out]
            n96 = call "Get NEW FI Set Max.vi"("error in (no error)"=w426) -> ("Error Out"=w425:errorcluster)  [unwired: 9 in, 1 out]
            n97 = call "FGV_GEA2_Ref.vi"("Action"=enum16{"Set Ref", "Get Ref"}."Get Ref", "Error In"=w425) -> ()  [unwired: 12 in, 2 out]
            n98 = Enqueue Element(queue=w429, element=T36 {"Data"=variant, "State"=enum."Init"} ("Data")) -> (error out=w430:errorcluster)  [unwired: 2 in, 2 out]
          }
          event Timeout {
            # "Must have timeout case to give GEA2 FGV a chance to update\nthe GEA2 reference. Otherwise, when we receive an event it may\nbe using a reference that is no longer valid."
            n99 = event-data() -> ()  [unwired: 1 in, 3 out]
          }
          event "Write ERD": Value Change {
            # "Read/Write ERDs Tab"
            n100 = event-data() -> ()  [unwired: 1 in, 1 out]
            n101 = call "GEA3 Write ERD (Rev 2 API) Multiple Messages.vi"("GEA2 Reference In"=w450, "# of Tries"=2 ("Retry Count"), "GEA Inputs"=w449, "Write ERD List"="Write ERD List", "Error In"=w447, "Verify ERD Response?"=TRUE) -> ("GEA2 Reference Out"=w451:refnum<k24>, "Error Out"=w446:errorcluster)  [unwired: 7 in, 1 out]
          }
          event "Read ERD": Value Change {
            # "Read/Write ERDs tab"
            n102 = event-data() -> ()  [unwired: 1 in, 6 out]
            n103 = call "GEA3 Read ERD (Rev 2 API) Multiple Messages.vi"("GEA2 Reference In"=w456, "Retry Count"=2, "GEA Inputs"=w455, "Read ERD List"="Read ERD List", "Error In"=w452, "Verify ERD Response?"=TRUE) -> ("GEA2 Reference Out"=w457:refnum<k24>, "ERD Data Out"=→"Read ERD Data Out":cluster{"ERD Number":u16, "Data":string}[], "Error Out"=w453:errorcluster)  [unwired: 6 in, 1 out]
          }
          event "UI Launch": Value Change {
            # "Main"
            n104 = event-data() -> ()  [unwired: 1 in, 6 out]
            n105 = call "HEUI_Running_FGV.vi"("Action"=enum16{"Get", "Set"}."Get", "Error In"=w467) -> ("Running?"=w464:bool, "Error Out"=w466:errorcluster)  [unwired: 12 in]
            n106 = Current VI's Path() -> (path=w462:path)
            n107 = Strip Path(path=w462) -> (stripped path=w463:path)  [unwired: 1 out]
            n108 = case shown="False" w464 {
              tunnel: w466 -> [w478 w480]
              tunnel: [w477 w480] -> w468
              tunnel: w463 -> [w470 _]
              tunnel: "UI Launch" -> [_ _]
              frame False {
                w479 = 128  # options
                n109 = Build Path(base path=w470, name or relative path="JLMainUI.vi") -> (appended path=w475:path)
                n110 = Open VI Reference(type specifier VI Refnum (for type only)=refnum<vi> refnum, vi path=w475, options=w479, error in (no error)=w478) -> (vi reference=w472:refnum<vi>, error out=w474:errorcluster)  [unwired: 2 in]
                n111 = call-by-ref "Start Asynchronous Call"(reference=w472, error in=w474) -> (reference out=w471:refnum<vi>, error out=w473:errorcluster)  [unwired: 10 in, 2 out]
                n112 = Close Reference(reference=w471, error in (no error)=w473) -> (error out=w477:errorcluster)
              }
              frame True {
              }
            }
          }
          event "Read Parametric": Value Change {
            # "Main"
            n113 = event-data() -> ()  [unwired: 1 in, 6 out]
            n114 = call "Para_ERD_Fxxx.vi"("GEA Inputs"=w485, "Error In"=w488, "Read ERD List"=T6[] [], "GEA2 Reference In"=w487) -> ("Error Out"=w482:errorcluster, "F6XX"=w483:T44, "GEA2 Reference Out"=w486:refnum<k24>)  [unwired: 4 in, 1 out]
            n115 = call "Parametric Viewer.vi"("Error In"=w482, "F6XX_In"=w483) -> ("Error Out"=w481:errorcluster)  [unwired: 8 in, 1 out]
          }
          event Value Change {
            (unwired) "ERD Loop" ("name (unnamed)")
            w495 = TRUE ("Blinking")
            # "GEA2 Tab"
            n116 = event-data() -> ()  [unwired: 1 in, 6 out]
            n117 = Generate User Event(user event=w499, event data cluster=TRUE ("event data"), error in=w502) -> (error out=w500:errorcluster)  [unwired: 1 in, 1 out]
            n118 = property on="Program Ind" class="Bool (strict)"(error in=w500, "Value"=w495, "Blinking"=w495) -> (error out=w496:errorcluster)  [unwired: 1 in, 1 out]
            n119 = Enqueue Element(queue=w493, element=T36 {"Data"=variant, "State"=enum."Pause"} ("Data"), error in (no error)=w496) -> (error out=w498:errorcluster)  [unwired: 1 in, 2 out]
            n120 = property on="GEA2 Send" class="Clust (strict)"() -> ("Value"=w491:T16)  [unwired: 2 in, 2 out]
            n121 = Unbundle By Name("Programming") -> ("File Path"=w506:path)
            n122 = call "Time Delay3"("error in (no error)"=w498, "Delay Time (s)"=2.0) -> ("error out"=w497:errorcluster)  [unwired: 9 in]
            n123 = Unbundle By Name(w491) -> ("Source"=w490:u8, "Destination"=w489:u8)
            n124 = Not Equal?(x=w506, y=path "") -> (x != y?=w505:bool)
            n125 = case shown="True" w505 {
              tunnel: w497 -> [w509 w514]
              tunnel: [w509 w521] -> w494
              tunnel: w506 -> [_ w526]
              tunnel: w503 -> [_ w522]
              tunnel: w490 -> [_ w511]
              tunnel: w489 -> [_ w510]
              frame False {
              }
              frame True {
                w512 = T15 9 items=["ImageRejected", "BoardNotFound", "UnableToGetGeaConfiguration", "WriteToFlashNotAllowed", "ImageDownloadedSuccessfully", "ImagePresent", "WriteToFlashFailed", "EraseFailed", "CrcFailed", ""] ("Result")
                w520 = FALSE ("Blinking")
                n126 = property on="Result" class="Ring (strict)"(error in=w514, "Value"=w512) -> (error out=w513:errorcluster)  [unwired: 1 in, 1 out]
                n127 = property on="Board Index" class="DigNum (strict)"(error in=w514, "DisabledEnum"=T39."Disabled and Grayed Out" ("Disabled")) -> ()  [unwired: 1 in, 2 out]
                n128 = call "GEA2 Flash APL.vi"("GEA2 Reference In"=w522, "Force Update?"=TRUE, "Source Address"=w511, "Destination Address"=w510, "File Path"=w526, "Error In"=w513, "Broadcast"=TRUE, "Reset?"=FALSE ("Reset Board?")) -> ("Result"=w515:i32, "Error Out"=w517:errorcluster)  [unwired: 3 in, 3 out]
                n129 = property on="Result" class="Ring (strict)"(error in=w517, "Value"=w515) -> (error out=w516:errorcluster)  [unwired: 1 in, 1 out]
                n130 = property on="Board Index" class="DigNum (strict)"(error in=w517, "DisabledEnum"=T39."Enabled" ("Disabled")) -> ()  [unwired: 1 in, 2 out]
                n131 = property on="Program Ind" class="Bool (strict)"(error in=w516, "Value"=w520, "Blinking"=w520) -> (error out=w521:errorcluster)  [unwired: 1 in, 1 out]
              }
            }
          }
          event "Flash Latest": Value Change {
            (unwired) "ERD Loop" ("name (unnamed)")
            w532 = TRUE ("Blinking")
            (unwired) FALSE ("Data On")
            # "GEA2 Tab"
            n132 = event-data() -> ()  [unwired: 1 in, 6 out]
            n133 = Generate User Event(user event=w541, event data cluster=TRUE ("event data"), error in=w542) -> (error out=w534:errorcluster)  [unwired: 1 in, 1 out]
            n134 = property on="Program Ind" class="Bool (strict)"(error in=w534, "Value"=w532, "Blinking"=w532) -> (error out=w533:errorcluster)  [unwired: 1 in, 1 out]
            n135 = Enqueue Element(queue=w538, element=T36 {"Data"=variant, "State"=enum."Pause"} ("Data"), error in (no error)=w533) -> (error out=w540:errorcluster)  [unwired: 1 in, 2 out]
            n136 = call "JL_Get_Latest_Build_From_Artifactory.vi"("Repository"="CIBuild") -> ("Output Path"=w527:path)  [unwired: 12 in, 2 out]
            n137 = call "Time Delay2"("error in (no error)"=w540, "Delay Time (s)"=3.0) -> ("error out"=w539:errorcluster)  [unwired: 9 in]
            n138 = Not Equal?(x=w527, y=path "") -> (x != y?=w545:bool)
            n139 = case shown="True" w545 {
              tunnel: w539 -> [w548 w572]
              tunnel: [w548 w560] -> w530
              tunnel: w543 -> [_ w573]
              tunnel: w527 -> [_ w549]
              frame False {
              }
              frame True {
                w552 = T15 9 items=["ImageRejected", "BoardNotFound", "UnableToGetGeaConfiguration", "WriteToFlashNotAllowed", "ImageDownloadedSuccessfully", "ImagePresent", "WriteToFlashFailed", "EraseFailed", "CrcFailed", ""] ("Result")
                w559 = FALSE ("Blinking")
                n140 = call "JL_APLPath.vi"("Error In"=w572, "APL Search String"=T40."UI Application APL", "Folder Path"=w549) -> ("Error Out"=w571:errorcluster, "File Path"=w570:path)  [unwired: 5 in, 2 out]
                n141 = call "GEA2 Flash APL.vi"("GEA2 Reference In"=w573, "Force Update?"=TRUE, "Source Address"=u8 228, "Destination Address"=u8 36, "File Path"=w570, "Error In"=w571, "Broadcast"=TRUE, "Reset?"=FALSE ("Reset Board?")) -> ("GEA2 Reference Out"=w562:refnum<k24>, "Result"=w556:i32, "Error Out"=w558:errorcluster)  [unwired: 3 in, 2 out]
                n142 = property on="Board Index" class="DigNum (strict)"(error in=w572, "DisabledEnum"=T39."Disabled and Grayed Out" ("Disabled")) -> (error out=w555:errorcluster)  [unwired: 1 in, 1 out]
                n143 = property on="Result" class="Ring (strict)"(error in=w558, "Value"=w556) -> (error out=w557:errorcluster)  [unwired: 1 in, 1 out]
                n144 = property on="Result" class="Ring (strict)"(error in=w555, "Value"=w552) -> ()  [unwired: 1 in, 2 out]
                n145 = call "JL_APLPath.vi"("Error In"=w557, "APL Search String"=T40."UI Parametric APL", "Folder Path"=w549) -> ("Error Out"=w568:errorcluster, "File Path"=w569:path)  [unwired: 5 in, 2 out]
                n146 = call "GEA2 Flash APL.vi"("GEA2 Reference In"=w562, "Force Update?"=TRUE, "Source Address"=u8 228, "Destination Address"=u8 36, "File Path"=w569, "Error In"=w568, "Broadcast"=TRUE, "Reset?"=TRUE ("Reset Board?")) -> ("Result"=w553:i32, "Error Out"=w561:errorcluster)  [unwired: 3 in, 3 out]
                n147 = property on="Board Index" class="DigNum (strict)"(error in=w561, "DisabledEnum"=T39."Enabled" ("Disabled")) -> (error out=w554:errorcluster)  [unwired: 1 in, 1 out]
                n148 = property on="Program Ind" class="Bool (strict)"(error in=w561, "Value"=w559, "Blinking"=w559) -> (error out=w560:errorcluster)  [unwired: 1 in, 1 out]
                n149 = property on="Result" class="Ring (strict)"(error in=w554, "Value"=w553) -> ()  [unwired: 1 in, 2 out]
              }
            }
            n150 = call "Time Delay4"("error in (no error)"=w530, "Delay Time (s)"=3.0) -> ("error out"=w529:errorcluster)  [unwired: 9 in]
            n151 = Enqueue Element(queue=w538, element=T36 {"Data"=variant, "State"=enum."Init"} ("Data"), error in (no error)=w529) -> (error out=w537:errorcluster)  [unwired: 1 in, 2 out]
          }
          event Value Change {
            # "GEA2 TAB"
            n152 = event-data() -> ()  [unwired: 1 in, 6 out]
            n153 = property on="GEA2 Send" class="Clust (strict)"() -> ("Value"=w584:T16)  [unwired: 2 in, 2 out]
            n154 = Unbundle By Name(w584) -> ("Source"=w583:u8)
            n155 = Bundle By Name(cluster=T16 {"Source"=228, "Destination"=36, "Command"=221, "Message"="F401"} ("Input Data"), "Source"=w583, "Destination"=u8 255, "Command"=u8 221, "Message"="F401") -> (w587:T16)
            n156 = call "GEA2 Send Message.vi"("GEA2 Reference In"=w594, "Input Data"=w587, "Error In"=w595) -> ("Error Out"=w581:errorcluster)  [unwired: 11 in, 1 out]
            n157 = call "Time Delay5"("error in (no error)"=w581, "Delay Time (s)"=3.0) -> ("error out"=w591:errorcluster)  [unwired: 9 in]
            n158 = Enqueue Element(queue=w589, element=T36 {"Data"=variant, "State"=enum."Init"} ("Data"), error in (no error)=w591) -> (error out=w590:errorcluster)  [unwired: 1 in, 2 out]
          }
          event Value Change {
            # "GEA2 Tab"
            n159 = event-data() -> ()  [unwired: 1 in, 6 out]
            n160 = property on="GEA2 Send" class="Clust (strict)"() -> ("Value"=w603:T16)  [unwired: 2 in, 2 out]
            n161 = Unbundle By Name(w603) -> ("Source"=w599:u8, "Destination"=w598:u8)
            n162 = Bundle By Name(cluster=T16 {"Source"=228, "Destination"=36, "Command"=221, "Message"="F401"} ("Input Data"), "Source"=w599, "Destination"=w598, "Command"=u8 221, "Message"="07") -> (w597:T16)
            n163 = call "GEA2 Send Message.vi"("GEA2 Reference In"=w605, "Input Data"=w597, "Error In"=w606) -> ("GEA2 Reference Out"=w604:refnum<k24>, "Error Out"=w596:errorcluster)  [unwired: 11 in]
          }
          event "Reset": Value Change {
            # "Main"
            n164 = event-data() -> ()  [unwired: 1 in, 6 out]
            n165 = call "GEA2 Write ERD.vi"("GEA2 Reference In"=w610, "GEA Inputs"=w609, "Write ERD List"=T7[] [{"ERD Number"=50, "Data Type"=enum."string", "Data"="01"}], "Error In"=w612) -> ("GEA2 Reference Out"=w608:refnum<k24>, "Error Out"=w607:errorcluster)  [unwired: 9 in, 1 out]
            n166 = Enqueue Element(queue=w613, element=T36 {"Data"=variant, "State"=enum."Init"} ("Data"), error in (no error)=w607) -> (error out=w614:errorcluster)  [unwired: 1 in, 2 out]
          }
          event "Save Log": Value Change {
            # "GEA2 Tab"
            n167 = event-data() -> ()  [unwired: 1 in, 6 out]
            n168 = property on="GEA2 Log" class="Str"(error in=w621) -> (error out=w623:errorcluster, "Value"=w622:string)  [unwired: 1 in, 1 out]
            n169 = Write to Text File(prompt (Choose or enter file path)="Choose filename and path to save txt file to ", text=w622, error in=w623) -> (refnum out=w620:refnum<file>, error out=w619:errorcluster)  [unwired: 1 in, 1 out]
            n170 = Close File(refnum=w620, error in=w619) -> (error out=w618:errorcluster)  [unwired: 1 out]
            n171 = call <vilib>:"Clear Errors.vi"("error in (no error)"=w618, "specific error code to clear (0: all)"=43) -> ("error out"=w617:errorcluster)  [unwired: 4 in, 1 out]
          }
          event "Run Script": Value Change {
            w652 = T24 {"Overall Script File Progress"=0.0, "Current Script Progress"=0.0, "Script"="", "Test"="", "Elapsed time (s)"=0.0, "Done?"=FALSE}  # Script Info
            w644 = T16 {"Source"=228, "Destination"=35, "Command"=1, "Message"=""}  # Version Query (for log header)
            # "Scripting Tab"
            n172 = event-data() -> ()  [unwired: 1 in, 6 out]
            n173 = Generate User Event(user event=w625, event data cluster=TRUE ("event data"), error in=w628) -> (error out=w629:errorcluster)  [unwired: 1 in, 1 out]
            n174 = Enqueue Element(queue=w626, element=T36 {"Data"=variant, "State"=enum."Pause"} ("Data"), error in (no error)=w629) -> (error out=w627:errorcluster)  [unwired: 1 in, 2 out]
            n175 = Obtain Queue(name (unnamed)="Script_Stop", element data type=FALSE, error in (no error)=w627) -> (queue out=w648:refnum<queue>, error out=w651:errorcluster)  [unwired: 2 in, 1 out]
            n176 = Obtain Queue(name (unnamed)="Script_Info", element data type=w652, error in (no error)=w651) -> (queue out=w654:refnum<queue>, error out=w645:errorcluster)  [unwired: 2 in, 1 out]
            n177 = while {
              tunnel: w654 -> [w666]
              shift-right: [w659] -> w642
              shift-left: w645 -> [w662]
              tunnel: [w665] -> w653
              tunnel: w648 -> [w663]
              tunnel: [w658] -> w646
              stop <- w664 stop-if-true
              n178 = Dequeue Element(queue=w666, error in (no error)=w662) -> (queue out=w665:refnum<queue>, element=w657:T24, error out=w661:errorcluster)  [unwired: 1 in, 1 out]
              "Script Info" <- w657
              n179 = Unbundle By Name(w657) -> ("Done?"=w664:bool)
              n180 = case shown="False" "stop script" {
                selector: "stop script" -> [_ w669]
                tunnel: w663 -> [w668 w673]
                tunnel: w662 -> [w667 w672]
                tunnel: [w667 w671] -> w660
                tunnel: [w668 w670] -> w658
                frame False {
                }
                frame True {
                  n181 = Enqueue Element(queue=w673, element=w669, error in (no error)=w672) -> (queue out=w670:refnum<queue>, error out=w671:errorcluster)  [unwired: 1 in, 1 out]
                }
              }
              n182 = Merge Errors(w660, w661) -> (w659:errorcluster)
            }
            n183 = call "GEA2 Script Test SLB.vi"("GEA2 Reference In"=w640, "Version Query (for log header)"=w644, "Enqueue Sends?"=TRUE, "Standalone"=FALSE, "Script path"="Script Path", "Log File Path (empty for prompt)"="Script Log Path", "Error In"=w645) -> ("Pass/Fail?"=→"Script Pass/Fail?":bool, "Report Text"=→"Script Report Text":string, "Error Out"=→"Script Error Out":errorcluster)  [unwired: 5 in, 1 out]
            n184 = Release Queue(queue=w653, error in (no error)=w642) -> (error out=w647:errorcluster)  [unwired: 1 in, 2 out]
            n185 = Release Queue(queue=w646, error in (no error)=w647) -> (error out=w632:errorcluster)  [unwired: 1 in, 2 out]
            n186 = Enqueue Element(queue=w626, element=T36 {"Data"=variant, "State"=enum."Init"} ("Data"), error in (no error)=w632) -> (error out=w631:errorcluster)  [unwired: 1 in, 2 out]
          }
          event Value Change {
            # "ERD List"
            n187 = event-data() -> ()  [unwired: 1 in, 6 out]
            n188 = Enqueue Element(queue=w676, element=T36 {"Data"=variant, "State"=enum."Build ERD Read List"}, error in (no error)=w678) -> (error out=w677:errorcluster)  [unwired: 1 in, 2 out]
            n189 = call "Write_Header_FGV.vi"("Write Header ? In"=TRUE, "Action"=enum16{"Get", "Set"}."Set", "Error In"=w677) -> ("Error Out"=w680:errorcluster)  [unwired: 11 in, 1 out]
            n190 = call "Select_List.vi"("Load ERD List"="Load ERD List") -> ()  [unwired: 14 in, 1 out]
          }
          event "Clear Fault Seq Buffer": Value Change {
            w696 = T7 {"ERD Number"=57626, "Data Type"=enum."string", "Data"=""}  # ERD Read Data In
            # "Faults Tab"
            n191 = event-data() -> ()  [unwired: 1 in, 6 out]
            n192 = Bundle By Name(cluster=w696, "Data"="01") -> (w695:T7)
            n193 = Build Array(w695) -> (w682:T7[])
            n194 = call "Convert Write ERD List to Message.vi"("GEA Inputs"=w684, "Write ERD List"=w682, "Error In"=w688) -> ("GEA Message"=w691:T16, "Error Out"=w692:errorcluster)  [unwired: 11 in]
            n195 = call "GEA2MessageFormatter.vi"("Prefix(Send/Recv)"="SEND", "GEA2 Data In"=w691, "Error In"=w692) -> ("Output String"=w693:string, "Error Out"=w694:errorcluster)  [unwired: 11 in]
            n196 = call "GExplorer_Queue_GEA2.vi"("Output String"=w693, "error in (no error)"=w694) -> ("error out"=w683:errorcluster)  [unwired: 13 in]
            n197 = call "GEA3 Write ERD (Rev 2 API) Multiple Messages.vi"("GEA2 Reference In"=w685, "GEA Inputs"=w684, "Write ERD List"=w682, "Error In"=w683) -> ("GEA2 Reference Out"=w686:refnum<k24>, "Error Out"=w687:errorcluster)  [unwired: 9 in, 1 out]
          }
          event "Get Faults": Value Change {
            # "Faults Tab"
            n198 = event-data() -> ()  [unwired: 1 in, 6 out]
            n199 = call "Main_Decode_V3.vi"("GEA2 Reference In"=w700, "GEA Inputs"=w704, "Error In"=w703) -> ("Fault Table Status"=w722:T19[], "Major Version"=→"Major Version":u8, "Minor Version"=→"Minor Version":u8, "Fault Table Entries"=w721:T20[][], "GEA2 Reference Out"=w711:refnum<k24>, "Diagnostic Entity Manifest"=w719:T21[], "SnapShot ERD List"=w709:T6[][], "Fault Sequence Status"=w712:T19[], "Fault Sequence Entries"=w720:T18[][], "Error Out"=w710:errorcluster)  [unwired: 5 in, 2 out]
            n200 = Index Array(array=w721) -> (element=w717:T20[])  [unwired: 2 in]
            n201 = Index Array(array=w722) -> (element=w698:T19)  [unwired: 1 in]
            "Fault Table Status" <- w698
            n202 = Index Array(array=w719) -> (element=→"Diagnostic Entity Manifest":T21)  [unwired: 1 in]
            n203 = Index Array(array=w720) -> (element=w714:T18[])  [unwired: 2 in]
            n204 = Index Array(array=w712) -> (element=w707:T19)  [unwired: 1 in]
            "Fault Seq Status" <- w707
            n205 = call "JL_Diag_Filter_Faults.vi"("Filter by Count"="Filter by Count", "Fault Table Entries In"=w717, "Status"=w698) -> ("Fault Table Entries Out"=→"Fault Table Entries":T20[], "Fault Set?"=→"Fault Set?":bool)  [unwired: 11 in]
            n206 = call "JL_Diag_Filter_Seq.vi"("Filter by Count"="Filter by Count", "Fault Table Entries In"=w714, "Status"=w707) -> ("Fault Table Entries Out"=→"Fault Sequence Entries":T18[])  [unwired: 12 in]
            n207 = Unbundle By Name(w698) -> ("Count"=w697:u16)
            n208 = Index Array(array=w709) -> (element=w708:T6[])  [unwired: 2 in]
            n209 = for {
              N: w697 -> [_]
              tunnel: [w731] -> w706 mode=indexing
              tunnel: w704 -> [w729]
              shift-right: [w728] -> w701
              shift-left: w711 -> [w730]
              shift-right: [w726] -> w702
              shift-left: w710 -> [w727]
              tunnel: w708 -> [w725] mode=indexing
              tunnel: "Filter by Count" -> [_]
              n210 = call "JL_Parse_Snapshot.vi"("GEA2 Reference In"=w730, "GEA Inputs"=w729, "SnapShot Location"=w725, "Error In"=w727) -> ("GEA2 Reference Out"=w728:refnum<k24>, "Fault Snapshot"=w731:string[], "Error Out"=w726:errorcluster)  [unwired: 9 in]
            }
            n211 = Transpose 2D Array(2D array=w706) -> (transposed array=→"Centauro Fault Snapshot":string[][])
          }
          event "Clear Fault Table Buffer": Value Change {
            # "Faults Tab"
            n212 = event-data() -> ()  [unwired: 1 in, 6 out]
            n213 = Bundle By Name(cluster=T7 {"ERD Number"=57604, "Data Type"=enum."string", "Data"=""} ("ERD Read Data In"), "Data"="01") -> (w741:T7)
            n214 = Build Array(w741) -> (w739:T7[])
            n215 = call "GEA3 Write ERD (Rev 2 API) Multiple Messages.vi"("GEA2 Reference In"=w738, "# of Tries"=u8 3, "Read Timeout (ms)"=u32 250, "GEA Inputs"=w737, "Write ERD List"=w739, "Error In"=w735) -> ("GEA2 Reference Out"=w736:refnum<k24>, "Error Out"=w734:errorcluster)  [unwired: 7 in, 1 out]
          }
          event "Get Cycle Data": Value Change {
            w743 = T6[] [{"ERD Number"=57661, "Data Type"=enum."string"}, {"ERD Number"=57662, "Data Type"=enum."string"}, {"ERD Number"=57663, "Data Type"=enum."string"}, {"ERD Number"=57664, "Data Type"=enum."string"}, {"ERD Number"=57665, "Data Type"=enum."string"}, {"ERD Number"=57666, "Data Type"=enum."string"}, {"ERD Number"=57667, "Data Type"=enum."string"}, {"ERD Number"=57668, "Data Type"=enum."string"}, {"ERD Number"=57669, "Data Type"=enum."string"}, {"ERD Number"=57670, "Data Type"=enum."string"}, {"ERD Number"=57671, "Data Type"=enum."string"}, {"ERD Number"=57672, "Data Type"=enum."string"}, {"ERD Number"=57673, "Data Type"=enum."string"}, {"ERD Number"=57674, "Data Type"=enum."string"}, {"ERD Number"=57675, "Data Type"=enum."string"}, {"ERD Number"=57676, "Data Type"=enum."string"}, {"ERD Number"=57677, "Data Type"=enum."string"}, {"ERD Number"=57678, "Data Type"=enum."string"}, {"ERD Number"=57679, "Data Type"=enum."string"}, {"ERD Number"=57680, "Data Type"=enum."string"}]
            # "E13D"
            # "Faults Tab"
            # "Erd_DiagnosticsCycleHistorySequenceEntry[0:19]"
            # "Erd_ServiceDiagnosticsCycleHistorySequenceStatus"
            n216 = event-data() -> ()  [unwired: 1 in, 1 out]
            n217 = call "GEA2 Read ERD.vi"("GEA2 Reference In"=w748, "GEA Inputs"=w751, "Read ERD List"=T6[] [{"ERD Number"=57659, "Data Type"=enum."string"}], "Error In"=w747) -> ("GEA2 Reference Out"=w753:refnum<k24>, "ERD Data Out"=w756:T9[], "Error Out"=w752:errorcluster)  [unwired: 8 in, 1 out]
            n218 = Index Array(array=w756) -> (element=w757:T9)  [unwired: 1 in]
            n219 = Unbundle By Name(w757) -> ("Data"=w767:string)
            n220 = call "HexStringToU16.vi"("Input String"=w767, "Starting Offset"=0) -> ("Number Out"=w765:u16)  [unwired: 13 in]
            n221 = call "HexStringToU16.vi"("Input String"=w767, "Starting Offset"=6) -> ("Number Out"=w768:u16)  [unwired: 13 in]
            n222 = call "HexStringToU16.vi"("Input String"=w767, "Starting Offset"=12) -> ("Number Out"=w766:u16)  [unwired: 13 in]
            n223 = Array Size(array=w743) -> (size(s)=w759:i32)
            n224 = Select(t=w768, s="Filter by Status Count", f=w759) -> (s? t:f=w758:i32)
            n225 = Bundle By Name(cluster=T19 {"Cur Index"=0, "Count"=0, "Ov Cnt"=0} ("Fault Table Status"), "Cur Index"=w765, "Count"=w768, "Ov Cnt"=w766) -> (→"output cluster":T19)
            n226 = Array Subset(array=w743, length=w758) -> (w755:T6[])  [unwired: 1 in]
            n227 = for {
              shift-right: [w774] -> w750
              shift-left: w752 -> [w775]
              shift-right: [w772] -> w749
              shift-left: w753 -> [w773]
              tunnel: w755 -> [w771] mode=indexing
              tunnel: w751 -> [w770]
              tunnel: [w769] -> w746 mode=indexing
              n228 = call "JL_Cycle_History_ParseRecord.vi"("Error In"=w775, "Cycle History ERD"=w771, "GEA Inputs"=w770, "GEA2 Reference In"=w773) -> ("Error Out"=w774:errorcluster, "CS2 Dryer"=w769:string[], "GEA2 Reference Out"=w772:refnum<k24>)  [unwired: 3 in, 1 out]
            }
            n229 = Transpose 2D Array(2D array=w746) -> (transposed array=→"JL Cycle History":string[][])
          }
          event "Data ON": Value Change {
            # "Main"
            n230 = event-data() -> ()  [unwired: 1 in, 6 out]
            n231 = case shown="True" "Data ON" {
              tunnel: w779 -> [w782 w786]
              tunnel: [w781 w785] -> w778
              tunnel: w776 -> [w780 w784]
              frame True {
                n232 = Enqueue Element(queue=w780, element=T36 {"Data"=variant, "State"=enum."Init"} ("Data"), error in (no error)=w782) -> (error out=w781:errorcluster)  [unwired: 1 in, 2 out]
              }
              frame False {
                n233 = Enqueue Element(queue=w784, element=T36 {"Data"=variant, "State"=enum."Pause"} ("Data"), error in (no error)=w786) -> (error out=w785:errorcluster)  [unwired: 1 in, 2 out]
              }
            }
          }
          event "Stop": Value Change; User Event; Panel Close {
            # "Main"
            n234 = event-data() -> ()  [unwired: 1 in, 3 out]
            n235 = call "Control_ERD_Loop.vi"("ERD Loop"=w788, "Command (ERD Loop Control)"=ERD_Loop_Control_Command."Shutdown", "Error In"=w797) -> ("Error Out"=w796:errorcluster)  [unwired: 12 in]
            n236 = call "Control_GEA2_Loop.vi"("Command (ERD Loop Control)"=GEA2_Control_Command."Shutdown", "Error In"=w796) -> ("Error Out"=w798:errorcluster)  [unwired: 13 in]
            n237 = call "Control_DAQ_Loop.vi"("Command (DAQ Control)"=DAQ_Control_Command."Shutdown", "Error In"=w798) -> ("Error Out"=w801:errorcluster)  [unwired: 13 in]
            n238 = call "Control_Cont_Send.vi"("Command (ERD Loop Control)"=GEA2_Control_Command."Shutdown", "Error In"=w801) -> ("Error Out"=w790:errorcluster)  [unwired: 13 in]
            n239 = call "Time Delay6"("error in (no error)"=w790, "Delay Time (s)"=1.0) -> ("error out"=w789:errorcluster)  [unwired: 9 in]
          }
          event "Tool Version": Value Change {
            # "Version Tab"
            n240 = event-data() -> ()  [unwired: 1 in, 6 out]
            n241 = property class="App"() -> ("App.Kind"=w804:T45)  [unwired: 2 in, 2 out]
            n242 = case shown="\"Run Time System\"" w804 {
              tunnel: ["invalid" ("File Version Info") w807 w812] -> w805
              frame "invalid app kind", Default {
              }
              frame "Development System", "Student Edition".."Evaluation" {
                n243 = property class="App"() -> ("App.Version"=w807:string)  [unwired: 2 in, 2 out]
              }
              frame "Run Time System" {
                n244 = property class="App"() -> ("App.Dir"=w810:path, "App.Name"=w811:string)  [unwired: 2 in, 2 out]
                n245 = Build Path(base path=w810, name or relative path=w811) -> (appended path=w809:path)
                n246 = call <vilib>:"FileVersionInfo.vi"("Application Path in"=w809) -> ("FileVersionInfo Out"=→"FileVersionInfo":T13, "File Version Info"=w812:string)  [unwired: 7 in, 2 out]
              }
            }
            "LabView/Version Number" <- w805
          }
          event "Get Wifi Data": Value Change {
            n247 = event-data() -> ()  [unwired: 1 in, 6 out]
            n248 = call "Wifi_Data.vi"("GEA2 Reference In"=w819, "Error In"=w820) -> ("Wifi Network State"=→"Wifi Network State":string, "GEA2 Reference Out"=w814:refnum<k24>, "Mac Address"=→"Mac Address":string, "Wifi Network Name"=→"Wifi Network Name":string, "Wifi Password"=→"Wifi Password":string, "Error Out"=w813:errorcluster)  [unwired: 8 in]
          }
          event "Turn off Wifi", "Turn on Wifi": Value Change {
            w822 = T7 {"ERD Number"=61717, "Data Type"=enum."string", "Data"=""} ("ERD Read Data In")
            n249 = event-data() -> ()  [unwired: 1 in, 6 out]
            n250 = case shown="True" "Turn on Wifi" {
              tunnel: w827 -> [w850 w857]
              tunnel: w826 -> [w851 w856]
              tunnel: w822 -> [_ w855]
              tunnel: [w851 w853] -> w824
              tunnel: [w850 w854] -> w825
              tunnel: w828 -> [w849 w852]
              tunnel: [w849 w852] -> w823
              frame False {
              }
              frame True {
                n251 = Concatenate Strings("01" ("string")) -> (w868:string)
                n252 = Bundle By Name(cluster=w855, "Data"=w868) -> (w867:T7)
                n253 = Build Array(w867) -> (w858:T7[])
                n254 = call "Convert Write ERD List to Message.vi"("GEA Inputs"=w852, "Write ERD List"=w858, "Error In"=w856) -> ("GEA Message"=w862:T16, "Error Out"=w863:errorcluster)  [unwired: 11 in]
                n255 = call "GEA2MessageFormatter.vi"("Prefix(Send/Recv)"="SEND", "GEA2 Data In"=w862, "Error In"=w863) -> ("Output String"=w864:string, "Error Out"=w865:errorcluster)  [unwired: 11 in]
                n256 = call "GExplorer_Queue_GEA2.vi"("Output String"=w864, "error in (no error)"=w865) -> ("error out"=w861:errorcluster)  [unwired: 13 in]
                n257 = call "GEA2 Write ERD.vi"("GEA2 Reference In"=w857, "GEA Inputs"=w852, "Write ERD List"=w858, "Error In"=w861, "Verify ERD Response?"=FALSE) -> ("GEA2 Reference Out"=w854:refnum<k24>, "Error Out"=w853:errorcluster)  [unwired: 8 in, 1 out]
              }
            }
            n258 = case shown="True" "Turn off Wifi" {
              tunnel: w825 -> [w830 w837]
              tunnel: w824 -> [w831 w836]
              tunnel: [w831 w834] -> _
              tunnel: [w830 w835] -> _
              tunnel: w823 -> [_ w833]
              tunnel: w822 -> [_ w832]
              frame False {
              }
              frame True {
                n259 = Concatenate Strings("02" ("string")) -> (w848:string)
                n260 = Bundle By Name(cluster=w832, "Data"=w848) -> (w847:T7)
                n261 = Build Array(w847) -> (w838:T7[])
                n262 = call "Convert Write ERD List to Message.vi"("GEA Inputs"=w833, "Write ERD List"=w838, "Error In"=w836) -> ("GEA Message"=w842:T16, "Error Out"=w843:errorcluster)  [unwired: 11 in]
                n263 = call "GEA2MessageFormatter.vi"("Prefix(Send/Recv)"="SEND", "GEA2 Data In"=w842, "Error In"=w843) -> ("Output String"=w844:string, "Error Out"=w845:errorcluster)  [unwired: 11 in]
                n264 = call "GExplorer_Queue_GEA2.vi"("Output String"=w844, "error in (no error)"=w845) -> ("error out"=w841:errorcluster)  [unwired: 13 in]
                n265 = call "GEA2 Write ERD.vi"("GEA2 Reference In"=w837, "GEA Inputs"=w833, "Write ERD List"=w838, "Error In"=w841, "Verify ERD Response?"=FALSE) -> ("GEA2 Reference Out"=w835:refnum<k24>, "Error Out"=w834:errorcluster)  [unwired: 8 in, 1 out]
              }
            }
          }
          event "EndOfCycle": Value Change {
            n266 = event-data() -> ()  [unwired: 1 in, 1 out]
            n267 = call "GEA2 Write ERD.vi"("GEA2 Reference In"=w874, "GEA Inputs"=w871, "Write ERD List"=T7[] [{"ERD Number"=61467, "Data Type"=enum."string", "Data"="05"}], "Error In"=w873) -> ("GEA2 Reference Out"=w870:refnum<k24>, "Error Out"=w869:errorcluster)  [unwired: 9 in, 1 out]
          }
          event "Set Wifi State(ERD 6003)": Value Change {
            n268 = event-data() -> ()  [unwired: 1 in, 6 out]
            n269 = case shown="\"0 - OFF\", Default" "Wifi State" {
              tunnel: ["00" "01" "02" "03" "04" "05" "06" "FF"] -> w881
              frame "0 - OFF", Default {
              }
              frame "1 - App Mode" {
              }
              frame "2 - Connecting" {
              }
              frame "3 - Connected" {
              }
              frame "4 - Connected Off" {
              }
              frame "5 - Scanning" {
              }
              frame "6 - Reconnecting" {
              }
              frame "255 - Invalid" {
              }
            }
            n270 = case shown="True" "Set Wifi State(ERD 6003)" {
              tunnel: w877 -> [w882 w887]
              tunnel: w878 -> [w883 w891]
              tunnel: [w883 w889] -> w876
              tunnel: [w882 w890] -> w875
              tunnel: w881 -> [_ w888]
              frame False {
              }
              frame True {
                w884 = T11 {"Source"=228, "Destination"=191} ("GEA Inputs")
                n271 = Concatenate Strings(w888) -> (w900:string)
                n272 = Bundle By Name(cluster=T7 {"ERD Number"=24579, "Data Type"=enum."string", "Data"=""} ("ERD Write Data In"), "Data"=w900) -> (w899:T7)
                n273 = Build Array(w899) -> (w885:T7[])
                n274 = call "Convert Write ERD List to Message.vi"("GEA Inputs"=w884, "Write ERD List"=w885, "Error In"=w891) -> ("GEA Message"=w895:T16, "Error Out"=w896:errorcluster)  [unwired: 11 in]
                n275 = call "GEA2MessageFormatter.vi"("Prefix(Send/Recv)"="SEND", "GEA2 Data In"=w895, "Error In"=w896) -> ("Output String"=w897:string, "Error Out"=w898:errorcluster)  [unwired: 11 in]
                n276 = call "GExplorer_Queue_GEA2.vi"("Output String"=w897, "error in (no error)"=w898) -> ("error out"=w894:errorcluster)  [unwired: 13 in]
                n277 = call "GEA2 Write ERD.vi"("GEA2 Reference In"=w887, "GEA Inputs"=w884, "Write ERD List"=w885, "Error In"=w894, "Verify ERD Response?"=FALSE) -> ("GEA2 Reference Out"=w890:refnum<k24>, "Error Out"=w889:errorcluster)  [unwired: 8 in, 1 out]
              }
            }
          }
        }
        n278 = call "Error_Control.vi"("Error In"=w351) -> ("Error Out"=w353:errorcluster)  [unwired: 14 in]
      }
      n279 = while "GEA2 Receive Message Loop" {
        shift-right: [w912] -> w91
        shift-left: w37 -> [w913]
        shift-right: [w909] -> _
        shift-left: w22 -> [w914]
        stop <- w911 stop-if-true
        # "GEA2 Receive Message Loop"
        n280 = event shown="[0] <Data_Recv>: User Event" {
          selector: w914 -> [w925 _ w948 w956 w974]
          dyn-events: [w925 _ w948 w957 w974] -> w909
          timeout: _ -> [_ _ _ _ _]
          tunnel: w913 -> [w922 w937 w940 w971 w976]
          tunnel: [w918 w937 w939 w958 w976] -> w910
          tunnel: [FALSE TRUE FALSE _ TRUE] -> w911
          event User Event {
            w928 = T16 {"Source"=0, "Destination"=0, "Command"=0, "Message"=""}  # GEA2 Data In
            # "Added subscription Ack"
            n281 = event-data() -> ("Source"=w927:u8, "Destination"=w924:u8, "Command"=w923:u8, "Message"=w916:string)  [unwired: 1 in]
            n282 = Bundle By Name(cluster=w928, "Source"=w927, "Destination"=w924, "Command"=w923, "Message"=w916) -> (w917:T16)
            n283 = call "GEA2 Log Filter.vi"("Filter Data"="Filter Data", "GEA2 Msg"=w917, "Cmd to ignore"="Ignore this CMD", "error in (no error)"=w922) -> ("error out"=w919:errorcluster)  [unwired: 11 in]
            n284 = property on="Program Ind" class="Bool (strict)"() -> ("Value"=w915:bool)  [unwired: 2 in, 2 out]
            n285 = case shown="False" w915 {
              tunnel: w919 -> [w934 w935]
              tunnel: [w932 w935] -> w918
              tunnel: w917 -> [w930 _]
              frame False {
                n286 = call "FGV_GEA2_Ref.vi"("Action"=enum16{"Set Ref", "Get Ref"}."Get Ref", "Error In"=w934) -> ("GEA2 Reference Out"=w931:refnum<k24>, "Error Out"=w933:errorcluster)  [unwired: 12 in]
                n287 = call "ACK Subscriptions Publications.vi"("GEA2 Reference In"=w931, "GEA2 Msg"=w930, "error in (no error)"=w933) -> ("error out"=w932:errorcluster)  [unwired: 11 in, 1 out]
              }
              frame True {
              }
            }
          }
          event User Event {
            n288 = event-data() -> ()  [unwired: 1 in, 7 out]
          }
          event User Event {
            # "This will update the UI with all data sent across the bus via a button Press"
            n289 = event-data() -> ("Source"=w950:T46, "Destination"=w947:u8, "Command"=w946:u8, "Message"=w945:string)  [unwired: 1 in]
            n290 = Bundle By Name(cluster=T16 {"Source"=0, "Destination"=0, "Command"=0, "Message"=""} ("GEA2 Data In"), "Source"=w950, "Destination"=w947, "Command"=w946, "Message"=w945) -> (w941:T16)
            n291 = property on="Program Ind" class="Bool (strict)"() -> ("Value"=w938:bool)  [unwired: 2 in, 2 out]
            n292 = call "GEA2MessageFormatter.vi"("Prefix(Send/Recv)"="SEND", "GEA2 Data In"=w941, "Error In"=w940) -> ("Output String"=w944:string, "Error Out"=w942:errorcluster)  [unwired: 11 in]
            n293 = case shown="False" w938 {
              tunnel: w944 -> [w954 _]
              tunnel: w942 -> [w953 w955]
              tunnel: [w952 w955] -> w939
              frame False {
                n294 = call "GExplorer_Queue_GEA2.vi"("Output String"=w954, "error in (no error)"=w953) -> ("error out"=w952:errorcluster)  [unwired: 13 in]
              }
              frame True {
              }
            }
          }
          event "Board Index": Value Change {
            # "Stop old GEA2\nbus reference"
            # "Allow other references a chance\nto begin using new reference"
            # "Store new GEA2 bus reference"
            # "Update event registration\nand initialize new GEA2 bus"
            # "Get the previous GEA2\nbus ref, but don't stop it\nuntil we update the FGV\nwith the new GEA2 ref"
            n295 = event-data() -> ("NewVal"=w968:u8)  [unwired: 1 in]
            n296 = property on="Board Index" class="DigNum (strict)"(error in=w971, "DisabledEnum"=T39."Disabled and Grayed Out" ("Disabled")) -> (error out=w972:errorcluster)  [unwired: 1 in, 1 out]
            n297 = call "FGV_GEA2_Ref.vi"("Action"=enum16{"Set Ref", "Get Ref"}."Get Ref", "Error In"=w972) -> ("GEA2 Reference Out"=w962:refnum<k24>, "Error Out"=w969:errorcluster)  [unwired: 12 in]
            n298 = call "GEA2_Reregister.vi"("Event Registration Refnum"=w956, "Board Index"=w968, "Error In"=w969) -> ("GEA2 Reference Out"=w967:refnum<k24>, "Event Registration Refnum 2"=w957:refnum<event-registration>, "Error Out"=w961:errorcluster)  [unwired: 9 in, 1 out]
            n299 = call "FGV_GEA2_Ref.vi"("GEA2 Reference In"=w967, "Action"=enum16{"Set Ref", "Get Ref"}."Set Ref", "Error In"=w961) -> ("Error Out"=w964:errorcluster)  [unwired: 11 in, 1 out]
            n300 = call "Time Delay"("error in (no error)"=w964, "Delay Time (s)"=5.0) -> ("error out"=w963:errorcluster)  [unwired: 9 in]
            n301 = call "GEA2 Stop.vi"("GEA2 Reference In"=w962, "Error In"=w963) -> ("Error Out"=w959:errorcluster)  [unwired: 13 in]
            n302 = property on="Board Index" class="DigNum (strict)"(error in=w959, "DisabledEnum"=T39."Enabled" ("Disabled")) -> (error out=w958:errorcluster)  [unwired: 1 in, 1 out]
          }
          event "Stop": Value Change {
            n303 = event-data() -> ()  [unwired: 1 in, 6 out]
          }
        }
        n304 = call "Error_Control.vi"("Error In"=w910) -> ("Error Out"=w912:errorcluster)  [unwired: 14 in]
      }
      n305 = while "Continuous Send Loop" {
        shift-right: [w104] -> _
        shift-left: Cont_Send_States."Run" ("State") -> [w103]
        tunnel: w50 -> [w105]
        tunnel: [w98] -> _
        shift-right: [w96] -> w53
        shift-left: w37 -> [w107]
        stop <- w106 stop-if-true
        # "Continuous Send Loop"
        n306 = Dequeue Element(queue=w105, timeout in ms (-1)=0, error in (no error)=w107) -> (queue out=w99:refnum<queue>, element=w92:T35, timed out?=w100:bool, error out=w95:errorcluster)
        n307 = Select(t=w103, s=w100, f=w92) -> (s? t:f=w102:T35)
        n308 = property on="GEA2 Send" class="Clust (strict)"() -> ("Value"=w94:T16)  [unwired: 2 in, 2 out]
        n309 = case shown="\"Shutdown\"" w102 {
          selector: w102 -> [w111 w122]
          tunnel: w95 -> [w113 w124]
          tunnel: [w112 w124] -> w97
          tunnel: [_ TRUE] -> w106
          tunnel: [w111 w122] -> w104
          tunnel: w99 -> [w110 w121]
          tunnel: [w110 w121] -> w98
          tunnel: w94 -> [w109 _]
          frame "Run", Default {
            n310 = case shown="True" "Start Send" {
              tunnel: w113 -> [w114 w117]
              tunnel: [w114 w120] -> w112
              tunnel: w109 -> [_ w119]
              frame False {
              }
              frame True {
                n311 = call "FGV_GEA2_Ref.vi"("Action"=enum16{"Set Ref", "Get Ref"}."Get Ref", "Error In"=w117) -> ("GEA2 Reference Out"=w116:refnum<k24>, "Error Out"=w115:errorcluster)  [unwired: 12 in]
                n312 = call "GEA2 Send Message.vi"("GEA2 Reference In"=w116, "Input Data"=w119, "Error In"=w115) -> ("Error Out"=w120:errorcluster)  [unwired: 11 in, 1 out]
              }
            }
          }
          frame "Shutdown" {
          }
        }
        n313 = call "Error_Control.vi"("Error In"=w97) -> ("Error Out"=w96:errorcluster)  [unwired: 14 in]
        n314 = Wait (ms)(milliseconds to wait="Msg Rate (ms)") -> ()  [unwired: 1 out]
      }
      n315 = while "GEA2 Display Loop" {
        tunnel: w38 -> [w309]
        shift-right: [w306] -> _
        shift-left: "" -> [w312]
        shift-right: [w308] -> w79
        shift-left: w47 -> [w316]
        tunnel: w45 -> [w302]
        tunnel: [w300] -> w43
        stop <- w310 stop-if-true
        # "Mensajes de los comandos enviados"
        # "GEA2 Display Loop"
        n316 = Dequeue Element(queue=w309, error in (no error)=w316) -> (element=w315:T38, error out=w311:errorcluster)  [unwired: 1 in, 2 out]
        n317 = Unbundle By Name(w315) -> ("Data"=w313:variant, "State"=w314:enum16{"Add to Log", "Clear", "Shutdown"})
        n318 = case shown="\"Add to Log\", Default" w314 {
          tunnel: w313 -> [w327 _ _]
          tunnel: w312 -> [w330 w335 _]
          tunnel: [w329 w335 ""] -> w307
          tunnel: w311 -> [w328 w336 w340]
          tunnel: [w325 w336 w340] -> w303
          tunnel: [FALSE TRUE FALSE] -> w310
          tunnel: [w317 _ _] -> w301
          frame "Add to Log", Default {
            n319 = Variant To Data(error in=w328, type="", Variant=w327) -> (data=w319:string, error out=w325:errorcluster)
            n320 = String Subset(string=w319, offset (0)=22, length (rest)=7 ("length (rest)")) -> (substring=w320:string)
            n321 = Equal?(x="SEND E5", y=w320) -> (x = y?=w318:bool)
            n322 = case shown="False" w318 {
              tunnel: w330 -> [w333 w334]
              tunnel: [w332 w334] -> w329
              tunnel: w319 -> [w331 _]
              tunnel: [w331 _] -> w317
              frame False {
                n323 = Concatenate Strings(w331, w333) -> (w332:string)
              }
              frame True {
              }
            }
          }
          frame "Shutdown" {
          }
          frame "Clear" {
          }
        }
        "GEA2 Log" <- w307
        n324 = call "Write _To_TXT_File.vi"("refnum"=w302, "text"=w301, "error in"=w303) -> ("refnum out"=w300:refnum<file>, "error out"=w304:errorcluster)  [unwired: 10 in, 1 out]
        n325 = String Subset(string=w307, length (rest)="GEA2 Log Length") -> (substring=w306:string)  [unwired: 1 in]
        n326 = call "Error_Control.vi"("Error In"=w304) -> ("Error Out"=w308:errorcluster)  [unwired: 14 in]
      }
      n327 = Close File(refnum=w43, error in=w79) -> (error out=w44:errorcluster)  [unwired: 1 out]
      n328 = call "GEA2 Stop.vi"("GEA2 Reference In"=w89, "Error In"=w90) -> ("Error Out"=w84:errorcluster)  [unwired: 13 in]
      n329 = Close File(refnum=w57, error in=w59) -> (error out=w58:errorcluster)  [unwired: 1 out]
      n330 = Merge Errors(w58, w44, w53, w91, w84) -> (w77:errorcluster)
      n331 = Obtain Queue(name (unnamed)="Continuous Send", element data type=Cont_Send_States."Run" ("State")) -> (queue out=w56:refnum<queue>, error out=w55:errorcluster)  [unwired: 3 in, 1 out]
      n332 = Obtain Queue(name (unnamed)="ERD Loop", element data type=T36 {"Data"=variant, "State"=enum."Read ERDs"} ("Data"), error in (no error)=w77) -> (queue out=w81:refnum<queue>, error out=w80:errorcluster)  [unwired: 2 in, 1 out]
      n333 = Obtain Queue(name (unnamed)="GEA2", element data type=T38 {"Data"=variant, "State"=enum."Add to Log"} ("Data"), error in (no error)=w77) -> (queue out=w88:refnum<queue>, error out=w87:errorcluster)  [unwired: 2 in, 1 out]
      n334 = Release Queue(queue=w56, error in (no error)=w55) -> (error out=w54:errorcluster)  [unwired: 1 in, 2 out]
      n335 = Release Queue(queue=w81, error in (no error)=w80) -> (error out=w75:errorcluster)  [unwired: 1 in, 2 out]
      n336 = Release Queue(queue=w88, error in (no error)=w87) -> (error out=w76:errorcluster)  [unwired: 1 in, 2 out]
      n337 = Merge Errors(w54, w75, w76) -> (w74:errorcluster)
      n338 = call "Error_Control.vi"("Command (Handle Errors)"=Error_Command."Report Errors", "Error In"=w74) -> ("Error Out"=w73:errorcluster)  [unwired: 13 in]
    }
    frame Error {
    }
  }
  n339 = call <vilib>:"Simple Error Handler.vi"("error in (no error)"=w15) -> ("error out"=→"Error Out":errorcluster)  [unwired: 4 in, 4 out]
